vi "ATS_Cards_GBL.vi"() -> ()   [LabVIEW 2010]
doc: "_____AlazarTech, Scope_____\n\nSPecifications of Cards and Pre-set value at Initialization.\n\nCards_Specs: array of specifications of card\n - Name: name of the card\n - Rate: text array of the possible clock rate of the card.\n - Range: text array of the possible input range of the card.\n\nCards_Pre-Set: array of pre-set value for each board."
uses:
  ATS_Card_Spec.ctl
  ATS_Global_4Ch.ctl
  Record.ctl
  Clock.ctl
  ClockSource.ctl
  ClockRate.ctl
  ClockEdge.ctl
  ATS_InputArray.ctl
  InputCtrl.ctl
  Coupling.ctl
  Range.ctl
  Impedance.ctl
  Bandwidth.ctl
  ATS_Trigger_4Ch.ctl
  TriggerOperation.ctl
  ATS_TriggerEngine_4Ch.ctl
  ATS_TriggerSource_4Ch.ctl
  ExtTrigger.ctl
  ExtTrigRange.ctl
  ATS_Global_Specs_Ctrl.ctl
panel:
  in  "Boards_Specs":cluster{"Name":string, "Specifications":T1}[](array[cluster])=[{"Name"="Unknown", "Specifications"={"ClckSource"={"Internal"=TRUE, "External"=TRUE, "Medium Ext."=FALSE, "Slow Ext."=FALSE, "Ext. AC"=FALSE, "Ext. DC"=FALSE, "Ext. (PLL)"=FALSE}, "ClckRate"={"1 kS/s"=TRUE, "2 kS/s"=TRUE, "5 kS/s"=TRUE, "10 kS/s"=TRUE, "20 kS/s"=TRUE, "50 kS/s"=TRUE, "100 kS/s"=TRUE, "200 kS/s"=TRUE, "500 kS/s"=TRUE, "1 MS/s"=TRUE, "2 MS/s"=TRUE, "5 MS/s"=TRUE, "10 MS/s"=TRUE, "20 MS/s"=TRUE, "25 MS/s"=TRUE, "50 MS/s"=TRUE, "100 MS/s"=TRUE, "125 MS/s"=FALSE, "160 MS/s"=FALSE, "180 MS/s"=FALSE, "200 MS/s"=TRUE, "250 MS/s"=FALSE, "500 MS/s"=TRUE, "1 GS/s"=TRUE}, "ClckEdge"={"Rising"=TRUE, "Falling"=TRUE}, "InputCoupling"={"AC"=TRUE, "DC"=TRUE}, "InputRange"={"20mV"=TRUE, "40mV"=TRUE, "50mV"=TRUE, "80mV"=TRUE, "100mV"=TRUE, "200mV"=TRUE, "400mV"=TRUE, "500mV"=TRUE, "800mV"=TRUE, "1 V"=TRUE, "2 V"=TRUE, "4 V"=TRUE, "5 V"=TRUE, "8 V"=TRUE, "10 V"=TRUE, "16 V"=FALSE, "20 V"=TRUE, "40 V"=FALSE, "HiFi"=FALSE, "1.25 V"=FALSE}, "Impedance"={"1M ohms"=TRUE, "50 ohms"=TRUE, "300 ohms"=FALSE}, "Bandwidth"={"Full"=TRUE, "Reduce"=FALSE}, "RangeLim(50)"="20 V", "AsyncDMA"={"OnBoard"=FALSE, "FPGA"=FALSE}, "Memory"={"VerifMem"=FALSE, "HighMem"=FALSE, "Combine"=FALSE, "HighRecord"=FALSE}, "ExtTrigCoupling"={"AC"=TRUE, "DC"=TRUE}, "ExtTrigRange"={"1 V"=TRUE, "5 V"=TRUE, "\nTTL"=FALSE}, "AUX_IO_Trig"={"Trig_Out"=FALSE, "Trig_In"=FALSE}, "AUX_IO_Slope"={"Rising"=FALSE, "Falling"=FALSE}, "MaxPretrig"={"MEM"=0, "FIFO"=0}, "AUX_I/O_Trig"={"OUT_Trigger"=FALSE, "OUT_PACER"=FALSE, "OUT_BUSY"=FALSE, "OUT_CLOCK"=FALSE, "OUT_RESERVED"=FALSE, "OUT_CAPTURE_ALMOST_DONE"=FALSE, "OUT_AUXILIARY"=FALSE, "OUT_SERIAL_DATA"=FALSE, "IN_TRIGGER_ENABLE"=FALSE, "IN_DIGITAL_TRIGGER"=FALSE, "IN_GATE"=FALSE, "IN_CAPTURE_ON_DEMAND"=FALSE, "IN_RESET_TIMESTAMP"=FALSE, "IN_SLOW_EXTERNAL_CLOCK"=FALSE, "INPUT_AUXILIARY"=FALSE, "INPUT_SERIAL_DATA"=FALSE}, "ChannelsPerBoard"=2}}, {"Name"="ATS850", "Specifications"={"ClckSource"={"Internal"=TRUE, "External"=TRUE, "Medium Ext."=FALSE, "Slow Ext."=FALSE, "Ext. AC"=FALSE, "Ext. DC"=FALSE, "Ext. (PLL)"=FALSE}, "ClckRate"={"1 kS/s"=TRUE, "2 kS/s"=TRUE, "5 kS/s"=TRUE, "10 kS/s"=TRUE, "20 kS/s"=TRUE, "50 kS/s"=TRUE, "100 kS/s"=TRUE, "200 kS/s"=TRUE, "500 kS/s"=TRUE, "1 MS/s"=TRUE, "2 MS/s"=TRUE, "5 MS/s"=TRUE, "10 MS/s"=TRUE, "20 MS/s"=FALSE, "25 MS/s"=TRUE, "50 MS/s"=TRUE, "100 MS/s"=FALSE, "125 MS/s"=FALSE, "160 MS/s"=FALSE, "180 MS/s"=FALSE, "200 MS/s"=FALSE, "250 MS/s"=FALSE, "500 MS/s"=FALSE, "1 GS/s"=FALSE}, "ClckEdge"={"Rising"=TRUE, "Falling"=TRUE}, "InputCoupling"={"AC"=TRUE, "DC"=TRUE}, "InputRange"={"20mV"=TRUE, "40mV"=TRUE, "50mV"=TRUE, "80mV"=TRUE, "100mV"=TRUE, "200mV"=TRUE, "400mV"=TRUE, "500mV"=TRUE, "800mV"=TRUE, "1 V"=TRUE, "2 V"=TRUE, "4 V"=TRUE, "5 V"=TRUE, "8 V"=TRUE, "10 V"=TRUE, "16 V"=FALSE, "20 V"=TRUE, "40 V"=FALSE, "HiFi"=FALSE, "1.25 V"=FALSE}, "Impedance"={"1M ohms"=TRUE, "50 ohms"=TRUE, "300 ohms"=FALSE}, "Bandwidth"={"Full"=TRUE, "Reduce"=FALSE}, "RangeLim(50)"="20 V", "AsyncDMA"={"OnBoard"=FALSE, "FPGA"=FALSE}, "Memory"={"VerifMem"=TRUE, "HighMem"=FALSE, "Combine"=FALSE, "HighRecord"=FALSE}, "ExtTrigCoupling"={"AC"=TRUE, "DC"=TRUE}, "ExtTrigRange"={"1 V"=TRUE, "5 V"=TRUE, "\nTTL"=FALSE}, "AUX_IO_Trig"={"Trig_Out"=FALSE, "Trig_In"=FALSE}, "AUX_IO_Slope"={"Rising"=FALSE, "Falling"=FALSE}, "MaxPretrig"={"MEM"=0, "FIFO"=0}, "AUX_I/O_Trig"={"OUT_Trigger"=FALSE, "OUT_PACER"=FALSE, "OUT_BUSY"=FALSE, "OUT_CLOCK"=FALSE, "OUT_RESERVED"=FALSE, "OUT_CAPTURE_ALMOST_DONE"=FALSE, "OUT_AUXILIARY"=FALSE, "OUT_SERIAL_DATA"=FALSE, "IN_TRIGGER_ENABLE"=FALSE, "IN_DIGITAL_TRIGGER"=FALSE, "IN_GATE"=FALSE, "IN_CAPTURE_ON_DEMAND"=FALSE, "IN_RESET_TIMESTAMP"=FALSE, "IN_SLOW_EXTERNAL_CLOCK"=FALSE, "INPUT_AUXILIARY"=FALSE, "INPUT_SERIAL_DATA"=FALSE}, "ChannelsPerBoard"=2}}, {"Name"="ATS310", "Specifications"={"ClckSource"={"Internal"=TRUE, "External"=TRUE, "Medium Ext."=FALSE, "Slow Ext."=FALSE, "Ext. AC"=FALSE, "Ext. DC"=FALSE, "Ext. (PLL)"=FALSE}, "ClckRate"={"1 kS/s"=TRUE, "2 kS/s"=TRUE, "5 kS/s"=TRUE, "10 kS/s"=TRUE, "20 kS/s"=TRUE, "50 kS/s"=TRUE, "100 kS/s"=TRUE, "200 kS/s"=TRUE, "500 kS/s"=TRUE, "1 MS/s"=TRUE, "2 MS/s"=TRUE, "5 MS/s"=TRUE, "10 MS/s"=TRUE, "20 MS/s"=TRUE, "25 MS/s"=FALSE, "50 MS/s"=FALSE, "100 MS/s"=FALSE, "125 MS/s"=FALSE, "160 MS/s"=FALSE, "180 MS/s"=FALSE, "200 MS/s"=FALSE, "250 MS/s"=FALSE, "500 MS/s"=FALSE, "1 GS/s"=FALSE}, "ClckEdge"={"Rising"=TRUE, "Falling"=TRUE}, "InputCoupling"={"AC"=TRUE, "DC"=TRUE}, "InputRange"={"20mV"=FALSE, "40mV"=TRUE, "50mV"=TRUE, "80mV"=TRUE, "100mV"=TRUE, "200mV"=TRUE, "400mV"=TRUE, "500mV"=TRUE, "800mV"=TRUE, "1 V"=TRUE, "2 V"=TRUE, "4 V"=TRUE, "5 V"=TRUE, "8 V"=TRUE, "10 V"=TRUE, "16 V"=FALSE, "20 V"=TRUE, "40 V"=FALSE, "HiFi"=FALSE, "1.25 V"=FALSE}, "Impedance"={"1M ohms"=TRUE, "50 ohms"=TRUE, "300 ohms"=FALSE}, "Bandwidth"={"Full"=TRUE, "Reduce"=FALSE}, "RangeLim(50)"="4 V", "AsyncDMA"={"OnBoard"=FALSE, "FPGA"=FALSE}, "Memory"={"VerifMem"=TRUE, "HighMem"=FALSE, "Combine"=FALSE, "HighRecord"=FALSE}, "ExtTrigCoupling"={"AC"=TRUE, "DC"=TRUE}, "ExtTrigRange"={"1 V"=TRUE, "5 V"=TRUE, "\nTTL"=FALSE}, "AUX_IO_Trig"={"Trig_Out"=FALSE, "Trig_In"=FALSE}, "AUX_IO_Slope"={"Rising"=FALSE, "Falling"=FALSE}, "MaxPretrig"={"MEM"=0, "FIFO"=0}, "AUX_I/O_Trig"={"OUT_Trigger"=FALSE, "OUT_PACER"=FALSE, "OUT_BUSY"=FALSE, "OUT_CLOCK"=FALSE, "OUT_RESERVED"=FALSE, "OUT_CAPTURE_ALMOST_DONE"=FALSE, "OUT_AUXILIARY"=FALSE, "OUT_SERIAL_DATA"=FALSE, "IN_TRIGGER_ENABLE"=FALSE, "IN_DIGITAL_TRIGGER"=FALSE, "IN_GATE"=FALSE, "IN_CAPTURE_ON_DEMAND"=FALSE, "IN_RESET_TIMESTAMP"=FALSE, "IN_SLOW_EXTERNAL_CLOCK"=FALSE, "INPUT_AUXILIARY"=FALSE, "INPUT_SERIAL_DATA"=FALSE}, "ChannelsPerBoard"=2}}, {"Name"="ATS330", "Specifications"={"ClckSource"={"Internal"=TRUE, "External"=TRUE, "Medium Ext."=FALSE, "Slow Ext."=FALSE, "Ext. AC"=FALSE, "Ext. DC"=FALSE, "Ext. (PLL)"=FALSE}, "ClckRate"={"1 kS/s"=TRUE, "2 kS/s"=TRUE, "5 kS/s"=TRUE, "10 kS/s"=TRUE, "20 kS/s"=TRUE, "50 kS/s"=TRUE, "100 kS/s"=TRUE, "200 kS/s"=TRUE, "500 kS/s"=TRUE, "1 MS/s"=TRUE, "2 MS/s"=TRUE, "5 MS/s"=TRUE, "10 MS/s"=TRUE, "20 MS/s"=FALSE, "25 MS/s"=TRUE, "50 MS/s"=TRUE, "100 MS/s"=FALSE, "125 MS/s"=FALSE, "160 MS/s"=FALSE, "180 MS/s"=FALSE, "200 MS/s"=FALSE, "250 MS/s"=FALSE, "500 MS/s"=FALSE, "1 GS/s"=FALSE}, "ClckEdge"={"Rising"=TRUE, "Falling"=TRUE}, "InputCoupling"={"AC"=TRUE, "DC"=TRUE}, "InputRange"={"20mV"=FALSE, "40mV"=TRUE, "50mV"=TRUE, "80mV"=TRUE, "100mV"=TRUE, "200mV"=TRUE, "400mV"=TRUE, "500mV"=TRUE, "800mV"=TRUE, "1 V"=TRUE, "2 V"=TRUE, "4 V"=TRUE, "5 V"=TRUE, "8 V"=TRUE, "10 V"=TRUE, "16 V"=FALSE, "20 V"=TRUE, "40 V"=FALSE, "HiFi"=FALSE, "1.25 V"=FALSE}, "Impedance"={"1M ohms"=TRUE, "50 ohms"=TRUE, "300 ohms"=FALSE}, "Bandwidth"={"Full"=TRUE, "Reduce"=FALSE}, "RangeLim(50)"="4 V", "AsyncDMA"={"OnBoard"=FALSE, "FPGA"=FALSE}, "Memory"={"VerifMem"=TRUE, "HighMem"=FALSE, "Combine"=FALSE, "HighRecord"=FALSE}, "ExtTrigCoupling"={"AC"=TRUE, "DC"=TRUE}, "ExtTrigRange"={"1 V"=TRUE, "5 V"=TRUE, "\nTTL"=FALSE}, "AUX_IO_Trig"={"Trig_Out"=FALSE, "Trig_In"=FALSE}, "AUX_IO_Slope"={"Rising"=FALSE, "Falling"=FALSE}, "MaxPretrig"={"MEM"=0, "FIFO"=0}, "AUX_I/O_Trig"={"OUT_Trigger"=FALSE, "OUT_PACER"=FALSE, "OUT_BUSY"=FALSE, "OUT_CLOCK"=FALSE, "OUT_RESERVED"=FALSE, "OUT_CAPTURE_ALMOST_DONE"=FALSE, "OUT_AUXILIARY"=FALSE, "OUT_SERIAL_DATA"=FALSE, "IN_TRIGGER_ENABLE"=FALSE, "IN_DIGITAL_TRIGGER"=FALSE, "IN_GATE"=FALSE, "IN_CAPTURE_ON_DEMAND"=FALSE, "IN_RESET_TIMESTAMP"=FALSE, "IN_SLOW_EXTERNAL_CLOCK"=FALSE, "INPUT_AUXILIARY"=FALSE, "INPUT_SERIAL_DATA"=FALSE}, "ChannelsPerBoard"=2}}, {"Name"="ATSxx4", "Specifications"={"ClckSource"={"Internal"=TRUE, "External"=TRUE, "Medium Ext."=FALSE, "Slow Ext."=FALSE, "Ext. AC"=FALSE, "Ext. DC"=FALSE, "Ext. (PLL)"=FALSE}, "ClckRate"={"1 kS/s"=TRUE, "2 kS/s"=TRUE, "5 kS/s"=TRUE, "10 kS/s"=TRUE, "20 kS/s"=TRUE, "50 kS/s"=TRUE, "100 kS/s"=TRUE, "200 kS/s"=TRUE, "500 kS/s"=TRUE, "1 MS/s"=TRUE, "2 MS/s"=TRUE, "5 MS/s"=TRUE, "10 MS/s"=TRUE, "20 MS/s"=TRUE, "25 MS/s"=TRUE, "50 MS/s"=TRUE, "100 MS/s"=TRUE, "125 MS/s"=FALSE, "160 MS/s"=FALSE, "180 MS/s"=FALSE, "200 MS/s"=TRUE, "250 MS/s"=FALSE, "500 MS/s"=TRUE, "1 GS/s"=TRUE}, "ClckEdge"={"Rising"=TRUE, "Falling"=TRUE}, "InputCoupling"={"AC"=TRUE, "DC"=TRUE}, "InputRange"={"20mV"=TRUE, "40mV"=TRUE, "50mV"=TRUE, "80mV"=TRUE, "100mV"=TRUE, "200mV"=TRUE, "400mV"=TRUE, "500mV"=TRUE, "800mV"=TRUE, "1 V"=TRUE, "2 V"=TRUE, "4 V"=TRUE, "5 V"=TRUE, "8 V"=TRUE, "10 V"=TRUE, "16 V"=FALSE, "20 V"=TRUE, "40 V"=FALSE, "HiFi"=FALSE, "1.25 V"=FALSE}, "Impedance"={"1M ohms"=TRUE, "50 ohms"=TRUE, "300 ohms"=FALSE}, "Bandwidth"={"Full"=TRUE, "Reduce"=FALSE}, "RangeLim(50)"="20 V", "AsyncDMA"={"OnBoard"=FALSE, "FPGA"=FALSE}, "Memory"={"VerifMem"=FALSE, "HighMem"=FALSE, "Combine"=FALSE, "HighRecord"=FALSE}, "ExtTrigCoupling"={"AC"=TRUE, "DC"=TRUE}, "ExtTrigRange"={"1 V"=TRUE, "5 V"=TRUE, "\nTTL"=FALSE}, "AUX_IO_Trig"={"Trig_Out"=FALSE, "Trig_In"=FALSE}, "AUX_IO_Slope"={"Rising"=FALSE, "Falling"=FALSE}, "MaxPretrig"={"MEM"=0, "FIFO"=0}, "AUX_I/O_Trig"={"OUT_Trigger"=FALSE, "OUT_PACER"=FALSE, "OUT_BUSY"=FALSE, "OUT_CLOCK"=FALSE, "OUT_RESERVED"=FALSE, "OUT_CAPTURE_ALMOST_DONE"=FALSE, "OUT_AUXILIARY"=FALSE, "OUT_SERIAL_DATA"=FALSE, "IN_TRIGGER_ENABLE"=FALSE, "IN_DIGITAL_TRIGGER"=FALSE, "IN_GATE"=FALSE, "IN_CAPTURE_ON_DEMAND"=FALSE, "IN_RESET_TIMESTAMP"=FALSE, "IN_SLOW_EXTERNAL_CLOCK"=FALSE, "INPUT_AUXILIARY"=FALSE, "INPUT_SERIAL_DATA"=FALSE}, "ChannelsPerBoard"=2}}, {"Name"="ATSxx5", "Specifications"={"ClckSource"={"Internal"=TRUE, "External"=TRUE, "Medium Ext."=FALSE, "Slow Ext."=FALSE, "Ext. AC"=FALSE, "Ext. DC"=FALSE, "Ext. (PLL)"=FALSE}, "ClckRate"={"1 kS/s"=TRUE, "2 kS/s"=TRUE, "5 kS/s"=TRUE, "10 kS/s"=TRUE, "20 kS/s"=TRUE, "50 kS/s"=TRUE, "100 kS/s"=TRUE, "200 kS/s"=TRUE, "500 kS/s"=TRUE, "1 MS/s"=TRUE, "2 MS/s"=TRUE, "5 MS/s"=TRUE, "10 MS/s"=TRUE, "20 MS/s"=TRUE, "25 MS/s"=TRUE, "50 MS/s"=TRUE, "100 MS/s"=TRUE, "125 MS/s"=FALSE, "160 MS/s"=FALSE, "180 MS/s"=FALSE, "200 MS/s"=TRUE, "250 MS/s"=FALSE, "500 MS/s"=TRUE, "1 GS/s"=TRUE}, "ClckEdge"={"Rising"=TRUE, "Falling"=TRUE}, "InputCoupling"={"AC"=TRUE, "DC"=TRUE}, "InputRange"={"20mV"=TRUE, "40mV"=TRUE, "50mV"=TRUE, "80mV"=TRUE, "100mV"=TRUE, "200mV"=TRUE, "400mV"=TRUE, "500mV"=TRUE, "800mV"=TRUE, "1 V"=TRUE, "2 V"=TRUE, "4 V"=TRUE, "5 V"=TRUE, "8 V"=TRUE, "10 V"=TRUE, "16 V"=FALSE, "20 V"=TRUE, "40 V"=FALSE, "HiFi"=FALSE, "1.25 V"=FALSE}, "Impedance"={"1M ohms"=TRUE, "50 ohms"=TRUE, "300 ohms"=FALSE}, "Bandwidth"={"Full"=TRUE, "Reduce"=FALSE}, "RangeLim(50)"="20 V", "AsyncDMA"={"OnBoard"=FALSE, "FPGA"=FALSE}, "Memory"={"VerifMem"=FALSE, "HighMem"=FALSE, "Combine"=FALSE, "HighRecord"=FALSE}, "ExtTrigCoupling"={"AC"=TRUE, "DC"=TRUE}, "ExtTrigRange"={"1 V"=TRUE, "5 V"=TRUE, "\nTTL"=FALSE}, "AUX_IO_Trig"={"Trig_Out"=FALSE, "Trig_In"=FALSE}, "AUX_IO_Slope"={"Rising"=FALSE, "Falling"=FALSE}, "MaxPretrig"={"MEM"=0, "FIFO"=0}, "AUX_I/O_Trig"={"OUT_Trigger"=FALSE, "OUT_PACER"=FALSE, "OUT_BUSY"=FALSE, "OUT_CLOCK"=FALSE, "OUT_RESERVED"=FALSE, "OUT_CAPTURE_ALMOST_DONE"=FALSE, "OUT_AUXILIARY"=FALSE, "OUT_SERIAL_DATA"=FALSE, "IN_TRIGGER_ENABLE"=FALSE, "IN_DIGITAL_TRIGGER"=FALSE, "IN_GATE"=FALSE, "IN_CAPTURE_ON_DEMAND"=FALSE, "IN_RESET_TIMESTAMP"=FALSE, "IN_SLOW_EXTERNAL_CLOCK"=FALSE, "INPUT_AUXILIARY"=FALSE, "INPUT_SERIAL_DATA"=FALSE}, "ChannelsPerBoard"=2}}, {"Name"="ATS460", "Specifications"={"ClckSource"={"Internal"=TRUE, "External"=TRUE, "Medium Ext."=TRUE, "Slow Ext."=TRUE, "Ext. AC"=FALSE, "Ext. DC"=FALSE, "Ext. (PLL)"=FALSE}, "ClckRate"={"1 kS/s"=FALSE, "2 kS/s"=FALSE, "5 kS/s"=FALSE, "10 kS/s"=TRUE, "20 kS/s"=TRUE, "50 kS/s"=TRUE, "100 kS/s"=TRUE, "200 kS/s"=TRUE, "500 kS/s"=TRUE, "1 MS/s"=TRUE, "2 MS/s"=TRUE, "5 MS/s"=TRUE, "10 MS/s"=TRUE, "20 MS/s"=TRUE, "25 MS/s"=FALSE, "50 MS/s"=TRUE, "100 MS/s"=TRUE, "125 MS/s"=TRUE, "160 MS/s"=FALSE, "180 MS/s"=FALSE, "200 MS/s"=FALSE, "250 MS/s"=FALSE, "500 MS/s"=FALSE, "1 GS/s"=FALSE}, "ClckEdge"={"Rising"=TRUE, "Falling"=TRUE}, "InputCoupling"={"AC"=TRUE, "DC"=TRUE}, "InputRange"={"20mV"=TRUE, "40mV"=TRUE, "50mV"=TRUE, "80mV"=TRUE, "100mV"=TRUE, "200mV"=TRUE, "400mV"=TRUE, "500mV"=TRUE, "800mV"=TRUE, "1 V"=TRUE, "2 V"=TRUE, "4 V"=TRUE, "5 V"=TRUE, "8 V"=TRUE, "10 V"=TRUE, "16 V"=FALSE, "20 V"=FALSE, "40 V"=FALSE, "HiFi"=TRUE, "1.25 V"=FALSE}, "Impedance"={"1M ohms"=TRUE, "50 ohms"=TRUE, "300 ohms"=FALSE}, "Bandwidth"={"Full"=TRUE, "Reduce"=TRUE}, "RangeLim(50)"="4 V", "AsyncDMA"={"OnBoard"=TRUE, "FPGA"=FALSE}, "Memory"={"VerifMem"=FALSE, "HighMem"=TRUE, "Combine"=FALSE, "HighRecord"=TRUE}, "ExtTrigCoupling"={"AC"=TRUE, "DC"=TRUE}, "ExtTrigRange"={"1 V"=TRUE, "5 V"=TRUE, "\nTTL"=FALSE}, "AUX_IO_Trig"={"Trig_Out"=FALSE, "Trig_In"=FALSE}, "AUX_IO_Slope"={"Rising"=FALSE, "Falling"=FALSE}, "MaxPretrig"={"MEM"=305419896, "FIFO"=0}, "AUX_I/O_Trig"={"OUT_Trigger"=FALSE, "OUT_PACER"=FALSE, "OUT_BUSY"=FALSE, "OUT_CLOCK"=FALSE, "OUT_RESERVED"=FALSE, "OUT_CAPTURE_ALMOST_DONE"=FALSE, "OUT_AUXILIARY"=FALSE, "OUT_SERIAL_DATA"=FALSE, "IN_TRIGGER_ENABLE"=FALSE, "IN_DIGITAL_TRIGGER"=FALSE, "IN_GATE"=FALSE, "IN_CAPTURE_ON_DEMAND"=FALSE, "IN_RESET_TIMESTAMP"=FALSE, "IN_SLOW_EXTERNAL_CLOCK"=FALSE, "INPUT_AUXILIARY"=FALSE, "INPUT_SERIAL_DATA"=FALSE}, "ChannelsPerBoard"=2}}, {"Name"="ATS660", "Specifications"={"ClckSource"={"Internal"=TRUE, "External"=TRUE, "Medium Ext."=FALSE, "Slow Ext."=TRUE, "Ext. AC"=TRUE, "Ext. DC"=TRUE, "Ext. (PLL)"=TRUE}, "ClckRate"={"1 kS/s"=TRUE, "2 kS/s"=TRUE, "5 kS/s"=TRUE, "10 kS/s"=TRUE, "20 kS/s"=TRUE, "50 kS/s"=TRUE, "100 kS/s"=TRUE, "200 kS/s"=TRUE, "500 kS/s"=TRUE, "1 MS/s"=TRUE, "2 MS/s"=TRUE, "5 MS/s"=TRUE, "10 MS/s"=TRUE, "20 MS/s"=TRUE, "25 MS/s"=FALSE, "50 MS/s"=TRUE, "100 MS/s"=TRUE, "125 MS/s"=TRUE, "160 MS/s"=FALSE, "180 MS/s"=FALSE, "200 MS/s"=FALSE, "250 MS/s"=FALSE, "500 MS/s"=FALSE, "1 GS/s"=FALSE}, "ClckEdge"={"Rising"=TRUE, "Falling"=TRUE}, "InputCoupling"={"AC"=TRUE, "DC"=TRUE}, "InputRange"={"20mV"=FALSE, "40mV"=FALSE, "50mV"=FALSE, "80mV"=FALSE, "100mV"=FALSE, "200mV"=TRUE, "400mV"=TRUE, "500mV"=FALSE, "800mV"=TRUE, "1 V"=FALSE, "2 V"=TRUE, "4 V"=TRUE, "5 V"=FALSE, "8 V"=TRUE, "10 V"=FALSE, "16 V"=TRUE, "20 V"=FALSE, "40 V"=FALSE, "HiFi"=FALSE, "1.25 V"=FALSE}, "Impedance"={"1M ohms"=TRUE, "50 ohms"=TRUE, "300 ohms"=FALSE}, "Bandwidth"={"Full"=TRUE, "Reduce"=TRUE}, "RangeLim(50)"="4 V", "AsyncDMA"={"OnBoard"=TRUE, "FPGA"=FALSE}, "Memory"={"VerifMem"=FALSE, "HighMem"=TRUE, "Combine"=FALSE, "HighRecord"=TRUE}, "ExtTrigCoupling"={"AC"=TRUE, "DC"=TRUE}, "ExtTrigRange"={"1 V"=TRUE, "5 V"=TRUE, "\nTTL"=FALSE}, "AUX_IO_Trig"={"Trig_Out"=FALSE, "Trig_In"=FALSE}, "AUX_IO_Slope"={"Rising"=FALSE, "Falling"=FALSE}, "MaxPretrig"={"MEM"=8386560, "FIFO"=0}, "AUX_I/O_Trig"={"OUT_Trigger"=FALSE, "OUT_PACER"=FALSE, "OUT_BUSY"=FALSE, "OUT_CLOCK"=FALSE, "OUT_RESERVED"=FALSE, "OUT_CAPTURE_ALMOST_DONE"=FALSE, "OUT_AUXILIARY"=FALSE, "OUT_SERIAL_DATA"=FALSE, "IN_TRIGGER_ENABLE"=FALSE, "IN_DIGITAL_TRIGGER"=FALSE, "IN_GATE"=FALSE, "IN_CAPTURE_ON_DEMAND"=FALSE, "IN_RESET_TIMESTAMP"=FALSE, "IN_SLOW_EXTERNAL_CLOCK"=FALSE, "INPUT_AUXILIARY"=FALSE, "INPUT_SERIAL_DATA"=FALSE}, "ChannelsPerBoard"=2}}, {"Name"="ATS860", "Specifications"={"ClckSource"={"Internal"=TRUE, "External"=TRUE, "Medium Ext."=FALSE, "Slow Ext."=FALSE, "Ext. AC"=FALSE, "Ext. DC"=FALSE, "Ext. (PLL)"=FALSE}, "ClckRate"={"1 kS/s"=TRUE, "2 kS/s"=TRUE, "5 kS/s"=TRUE, "10 kS/s"=TRUE, "20 kS/s"=TRUE, "50 kS/s"=TRUE, "100 kS/s"=TRUE, "200 kS/s"=TRUE, "500 kS/s"=TRUE, "1 MS/s"=TRUE, "2 MS/s"=TRUE, "5 MS/s"=TRUE, "10 MS/s"=TRUE, "20 MS/s"=FALSE, "25 MS/s"=TRUE, "50 MS/s"=TRUE, "100 MS/s"=FALSE, "125 MS/s"=TRUE, "160 MS/s"=FALSE, "180 MS/s"=FALSE, "200 MS/s"=FALSE, "250 MS/s"=TRUE, "500 MS/s"=FALSE, "1 GS/s"=FALSE}, "ClckEdge"={"Rising"=TRUE, "Falling"=TRUE}, "InputCoupling"={"AC"=TRUE, "DC"=TRUE}, "InputRange"={"20mV"=TRUE, "40mV"=TRUE, "50mV"=TRUE, "80mV"=TRUE, "100mV"=TRUE, "200mV"=TRUE, "400mV"=TRUE, "500mV"=TRUE, "800mV"=TRUE, "1 V"=TRUE, "2 V"=TRUE, "4 V"=TRUE, "5 V"=TRUE, "8 V"=TRUE, "10 V"=TRUE, "16 V"=FALSE, "20 V"=FALSE, "40 V"=FALSE, "HiFi"=FALSE, "1.25 V"=FALSE}, "Impedance"={"1M ohms"=TRUE, "50 ohms"=TRUE, "300 ohms"=FALSE}, "Bandwidth"={"Full"=TRUE, "Reduce"=TRUE}, "RangeLim(50)"="4 V", "AsyncDMA"={"OnBoard"=TRUE, "FPGA"=FALSE}, "Memory"={"VerifMem"=FALSE, "HighMem"=TRUE, "Combine"=FALSE, "HighRecord"=TRUE}, "ExtTrigCoupling"={"AC"=TRUE, "DC"=TRUE}, "ExtTrigRange"={"1 V"=TRUE, "5 V"=TRUE, "\nTTL"=FALSE}, "AUX_IO_Trig"={"Trig_Out"=FALSE, "Trig_In"=FALSE}, "AUX_IO_Slope"={"Rising"=FALSE, "Falling"=FALSE}, "MaxPretrig"={"MEM"=0, "FIFO"=0}, "AUX_I/O_Trig"={"OUT_Trigger"=FALSE, "OUT_PACER"=FALSE, "OUT_BUSY"=FALSE, "OUT_CLOCK"=FALSE, "OUT_RESERVED"=FALSE, "OUT_CAPTURE_ALMOST_DONE"=FALSE, "OUT_AUXILIARY"=FALSE, "OUT_SERIAL_DATA"=FALSE, "IN_TRIGGER_ENABLE"=FALSE, "IN_DIGITAL_TRIGGER"=FALSE, "IN_GATE"=FALSE, "IN_CAPTURE_ON_DEMAND"=FALSE, "IN_RESET_TIMESTAMP"=FALSE, "IN_SLOW_EXTERNAL_CLOCK"=FALSE, "INPUT_AUXILIARY"=FALSE, "INPUT_SERIAL_DATA"=FALSE}, "ChannelsPerBoard"=2}}, {"Name"="Unknown", "Specifications"={"ClckSource"={"Internal"=TRUE, "External"=TRUE, "Medium Ext."=FALSE, "Slow Ext."=FALSE, "Ext. AC"=FALSE, "Ext. DC"=FALSE, "Ext. (PLL)"=FALSE}, "ClckRate"={"1 kS/s"=TRUE, "2 kS/s"=TRUE, "5 kS/s"=TRUE, "10 kS/s"=TRUE, "20 kS/s"=TRUE, "50 kS/s"=TRUE, "100 kS/s"=TRUE, "200 kS/s"=TRUE, "500 kS/s"=TRUE, "1 MS/s"=TRUE, "2 MS/s"=TRUE, "5 MS/s"=TRUE, "10 MS/s"=TRUE, "20 MS/s"=TRUE, "25 MS/s"=FALSE, "50 MS/s"=TRUE, "100 MS/s"=TRUE, "125 MS/s"=TRUE, "160 MS/s"=FALSE, "180 MS/s"=FALSE, "200 MS/s"=FALSE, "250 MS/s"=FALSE, "500 MS/s"=FALSE, "1 GS/s"=FALSE}, "ClckEdge"={"Rising"=TRUE, "Falling"=TRUE}, "InputCoupling"={"AC"=TRUE, "DC"=TRUE}, "InputRange"={"20mV"=FALSE, "40mV"=FALSE, "50mV"=FALSE, "80mV"=FALSE, "100mV"=FALSE, "200mV"=TRUE, "400mV"=TRUE, "500mV"=FALSE, "800mV"=TRUE, "1 V"=FALSE, "2 V"=TRUE, "4 V"=TRUE, "5 V"=FALSE, "8 V"=TRUE, "10 V"=FALSE, "16 V"=TRUE, "20 V"=FALSE, "40 V"=FALSE, "HiFi"=FALSE, "1.25 V"=FALSE}, "Impedance"={"1M ohms"=TRUE, "50 ohms"=TRUE, "300 ohms"=FALSE}, "Bandwidth"={"Full"=TRUE, "Reduce"=TRUE}, "RangeLim(50)"="4 V", "AsyncDMA"={"OnBoard"=FALSE, "FPGA"=FALSE}, "Memory"={"VerifMem"=FALSE, "HighMem"=FALSE, "Combine"=FALSE, "HighRecord"=FALSE}, "ExtTrigCoupling"={"AC"=TRUE, "DC"=TRUE}, "ExtTrigRange"={"1 V"=TRUE, "5 V"=TRUE, "\nTTL"=FALSE}, "AUX_IO_Trig"={"Trig_Out"=FALSE, "Trig_In"=FALSE}, "AUX_IO_Slope"={"Rising"=FALSE, "Falling"=FALSE}, "MaxPretrig"={"MEM"=0, "FIFO"=0}, "AUX_I/O_Trig"={"OUT_Trigger"=FALSE, "OUT_PACER"=FALSE, "OUT_BUSY"=FALSE, "OUT_CLOCK"=FALSE, "OUT_RESERVED"=FALSE, "OUT_CAPTURE_ALMOST_DONE"=FALSE, "OUT_AUXILIARY"=FALSE, "OUT_SERIAL_DATA"=FALSE, "IN_TRIGGER_ENABLE"=FALSE, "IN_DIGITAL_TRIGGER"=FALSE, "IN_GATE"=FALSE, "IN_CAPTURE_ON_DEMAND"=FALSE, "IN_RESET_TIMESTAMP"=FALSE, "IN_SLOW_EXTERNAL_CLOCK"=FALSE, "INPUT_AUXILIARY"=FALSE, "INPUT_SERIAL_DATA"=FALSE}, "ChannelsPerBoard"=2}}, {"Name"="Unknown", "Specifications"={"ClckSource"={"Internal"=TRUE, "External"=TRUE, "Medium Ext."=FALSE, "Slow Ext."=FALSE, "Ext. AC"=FALSE, "Ext. DC"=FALSE, "Ext. (PLL)"=FALSE}, "ClckRate"={"1 kS/s"=TRUE, "2 kS/s"=TRUE, "5 kS/s"=TRUE, "10 kS/s"=TRUE, "20 kS/s"=TRUE, "50 kS/s"=TRUE, "100 kS/s"=TRUE, "200 kS/s"=TRUE, "500 kS/s"=TRUE, "1 MS/s"=TRUE, "2 MS/s"=TRUE, "5 MS/s"=TRUE, "10 MS/s"=TRUE, "20 MS/s"=TRUE, "25 MS/s"=FALSE, "50 MS/s"=TRUE, "100 MS/s"=TRUE, "125 MS/s"=TRUE, "160 MS/s"=FALSE, "180 MS/s"=FALSE, "200 MS/s"=FALSE, "250 MS/s"=FALSE, "500 MS/s"=FALSE, "1 GS/s"=FALSE}, "ClckEdge"={"Rising"=TRUE, "Falling"=TRUE}, "InputCoupling"={"AC"=TRUE, "DC"=TRUE}, "InputRange"={"20mV"=FALSE, "40mV"=FALSE, "50mV"=FALSE, "80mV"=FALSE, "100mV"=FALSE, "200mV"=TRUE, "400mV"=TRUE, "500mV"=FALSE, "800mV"=TRUE, "1 V"=FALSE, "2 V"=TRUE, "4 V"=TRUE, "5 V"=FALSE, "8 V"=TRUE, "10 V"=FALSE, "16 V"=TRUE, "20 V"=FALSE, "40 V"=FALSE, "HiFi"=FALSE, "1.25 V"=FALSE}, "Impedance"={"1M ohms"=TRUE, "50 ohms"=TRUE, "300 ohms"=FALSE}, "Bandwidth"={"Full"=TRUE, "Reduce"=TRUE}, "RangeLim(50)"="4 V", "AsyncDMA"={"OnBoard"=FALSE, "FPGA"=FALSE}, "Memory"={"VerifMem"=FALSE, "HighMem"=FALSE, "Combine"=FALSE, "HighRecord"=FALSE}, "ExtTrigCoupling"={"AC"=TRUE, "DC"=TRUE}, "ExtTrigRange"={"1 V"=TRUE, "5 V"=TRUE, "\nTTL"=FALSE}, "AUX_IO_Trig"={"Trig_Out"=FALSE, "Trig_In"=FALSE}, "AUX_IO_Slope"={"Rising"=FALSE, "Falling"=FALSE}, "MaxPretrig"={"MEM"=0, "FIFO"=0}, "AUX_I/O_Trig"={"OUT_Trigger"=FALSE, "OUT_PACER"=FALSE, "OUT_BUSY"=FALSE, "OUT_CLOCK"=FALSE, "OUT_RESERVED"=FALSE, "OUT_CAPTURE_ALMOST_DONE"=FALSE, "OUT_AUXILIARY"=FALSE, "OUT_SERIAL_DATA"=FALSE, "IN_TRIGGER_ENABLE"=FALSE, "IN_DIGITAL_TRIGGER"=FALSE, "IN_GATE"=FALSE, "IN_CAPTURE_ON_DEMAND"=FALSE, "IN_RESET_TIMESTAMP"=FALSE, "IN_SLOW_EXTERNAL_CLOCK"=FALSE, "INPUT_AUXILIARY"=FALSE, "INPUT_SERIAL_DATA"=FALSE}, "ChannelsPerBoard"=2}}, {"Name"="ATS9462", "Specifications"={"ClckSource"={"Internal"=TRUE, "External"=TRUE, "Medium Ext."=FALSE, "Slow Ext."=TRUE, "Ext. AC"=FALSE, "Ext. DC"=TRUE, "Ext. (PLL)"=TRUE}, "ClckRate"={"1 kS/s"=TRUE, "2 kS/s"=TRUE, "5 kS/s"=TRUE, "10 kS/s"=TRUE, "20 kS/s"=TRUE, "50 kS/s"=TRUE, "100 kS/s"=TRUE, "200 kS/s"=TRUE, "500 kS/s"=TRUE, "1 MS/s"=TRUE, "2 MS/s"=TRUE, "5 MS/s"=TRUE, "10 MS/s"=TRUE, "20 MS/s"=TRUE, "25 MS/s"=FALSE, "50 MS/s"=TRUE, "100 MS/s"=TRUE, "125 MS/s"=TRUE, "160 MS/s"=TRUE, "180 MS/s"=TRUE, "200 MS/s"=FALSE, "250 MS/s"=FALSE, "500 MS/s"=FALSE, "1 GS/s"=FALSE}, "ClckEdge"={"Rising"=TRUE, "Falling"=TRUE}, "InputCoupling"={"AC"=TRUE, "DC"=TRUE}, "InputRange"={"20mV"=FALSE, "40mV"=FALSE, "50mV"=FALSE, "80mV"=FALSE, "100mV"=FALSE, "200mV"=TRUE, "400mV"=TRUE, "500mV"=FALSE, "800mV"=TRUE, "1 V"=FALSE, "2 V"=TRUE, "4 V"=TRUE, "5 V"=FALSE, "8 V"=TRUE, "10 V"=FALSE, "16 V"=TRUE, "20 V"=FALSE, "40 V"=FALSE, "HiFi"=FALSE, "1.25 V"=FALSE}, "Impedance"={"1M ohms"=TRUE, "50 ohms"=TRUE, "300 ohms"=FALSE}, "Bandwidth"={"Full"=TRUE, "Reduce"=TRUE}, "RangeLim(50)"="4 V", "AsyncDMA"={"OnBoard"=TRUE, "FPGA"=TRUE}, "Memory"={"VerifMem"=FALSE, "HighMem"=TRUE, "Combine"=FALSE, "HighRecord"=TRUE}, "ExtTrigCoupling"={"AC"=TRUE, "DC"=TRUE}, "ExtTrigRange"={"1 V"=TRUE, "5 V"=TRUE, "\nTTL"=FALSE}, "AUX_IO_Trig"={"Trig_Out"=TRUE, "Trig_In"=TRUE}, "AUX_IO_Slope"={"Rising"=TRUE, "Falling"=TRUE}, "MaxPretrig"={"MEM"=0, "FIFO"=0}, "AUX_I/O_Trig"={"OUT_Trigger"=TRUE, "OUT_PACER"=FALSE, "OUT_BUSY"=FALSE, "OUT_CLOCK"=FALSE, "OUT_RESERVED"=FALSE, "OUT_CAPTURE_ALMOST_DONE"=FALSE, "OUT_AUXILIARY"=FALSE, "OUT_SERIAL_DATA"=FALSE, "IN_TRIGGER_ENABLE"=TRUE, "IN_DIGITAL_TRIGGER"=TRUE, "IN_GATE"=FALSE, "IN_CAPTURE_ON_DEMAND"=FALSE, "IN_RESET_TIMESTAMP"=FALSE, "IN_SLOW_EXTERNAL_CLOCK"=FALSE, "INPUT_AUXILIARY"=FALSE, "INPUT_SERIAL_DATA"=FALSE}, "ChannelsPerBoard"=2}}, {"Name"="Unknown", "Specifications"={"ClckSource"={"Internal"=TRUE, "External"=TRUE, "Medium Ext."=FALSE, "Slow Ext."=FALSE, "Ext. AC"=FALSE, "Ext. DC"=FALSE, "Ext. (PLL)"=FALSE}, "ClckRate"={"1 kS/s"=TRUE, "2 kS/s"=TRUE, "5 kS/s"=TRUE, "10 kS/s"=TRUE, "20 kS/s"=TRUE, "50 kS/s"=TRUE, "100 kS/s"=TRUE, "200 kS/s"=TRUE, "500 kS/s"=TRUE, "1 MS/s"=TRUE, "2 MS/s"=TRUE, "5 MS/s"=TRUE, "10 MS/s"=TRUE, "20 MS/s"=TRUE, "25 MS/s"=FALSE, "50 MS/s"=TRUE, "100 MS/s"=TRUE, "125 MS/s"=TRUE, "160 MS/s"=FALSE, "180 MS/s"=FALSE, "200 MS/s"=FALSE, "250 MS/s"=FALSE, "500 MS/s"=FALSE, "1 GS/s"=FALSE}, "ClckEdge"={"Rising"=TRUE, "Falling"=TRUE}, "InputCoupling"={"AC"=TRUE, "DC"=TRUE}, "InputRange"={"20mV"=FALSE, "40mV"=FALSE, "50mV"=FALSE, "80mV"=FALSE, "100mV"=FALSE, "200mV"=TRUE, "400mV"=TRUE, "500mV"=FALSE, "800mV"=TRUE, "1 V"=FALSE, "2 V"=TRUE, "4 V"=TRUE, "5 V"=FALSE, "8 V"=TRUE, "10 V"=FALSE, "16 V"=TRUE, "20 V"=FALSE, "40 V"=FALSE, "HiFi"=FALSE, "1.25 V"=FALSE}, "Impedance"={"1M ohms"=TRUE, "50 ohms"=TRUE, "300 ohms"=FALSE}, "Bandwidth"={"Full"=TRUE, "Reduce"=TRUE}, "RangeLim(50)"="4 V", "AsyncDMA"={"OnBoard"=FALSE, "FPGA"=FALSE}, "Memory"={"VerifMem"=FALSE, "HighMem"=FALSE, "Combine"=FALSE, "HighRecord"=FALSE}, "ExtTrigCoupling"={"AC"=TRUE, "DC"=TRUE}, "ExtTrigRange"={"1 V"=TRUE, "5 V"=TRUE, "\nTTL"=FALSE}, "AUX_IO_Trig"={"Trig_Out"=FALSE, "Trig_In"=FALSE}, "AUX_IO_Slope"={"Rising"=FALSE, "Falling"=FALSE}, "MaxPretrig"={"MEM"=0, "FIFO"=0}, "AUX_I/O_Trig"={"OUT_Trigger"=FALSE, "OUT_PACER"=FALSE, "OUT_BUSY"=FALSE, "OUT_CLOCK"=FALSE, "OUT_RESERVED"=FALSE, "OUT_CAPTURE_ALMOST_DONE"=FALSE, "OUT_AUXILIARY"=FALSE, "OUT_SERIAL_DATA"=FALSE, "IN_TRIGGER_ENABLE"=FALSE, "IN_DIGITAL_TRIGGER"=FALSE, "IN_GATE"=FALSE, "IN_CAPTURE_ON_DEMAND"=FALSE, "IN_RESET_TIMESTAMP"=FALSE, "IN_SLOW_EXTERNAL_CLOCK"=FALSE, "INPUT_AUXILIARY"=FALSE, "INPUT_SERIAL_DATA"=FALSE}, "ChannelsPerBoard"=2}}, {"Name"="ATS9870", "Specifications"={"ClckSource"={"Internal"=TRUE, "External"=TRUE, "Medium Ext."=FALSE, "Slow Ext."=FALSE, "Ext. AC"=TRUE, "Ext. DC"=TRUE, "Ext. (PLL)"=TRUE}, "ClckRate"={"1 kS/s"=TRUE, "2 kS/s"=TRUE, "5 kS/s"=TRUE, "10 kS/s"=TRUE, "20 kS/s"=TRUE, "50 kS/s"=TRUE, "100 kS/s"=TRUE, "200 kS/s"=TRUE, "500 kS/s"=TRUE, "1 MS/s"=TRUE, "2 MS/s"=TRUE, "5 MS/s"=TRUE, "10 MS/s"=TRUE, "20 MS/s"=TRUE, "25 MS/s"=FALSE, "50 MS/s"=TRUE, "100 MS/s"=TRUE, "125 MS/s"=FALSE, "160 MS/s"=FALSE, "180 MS/s"=FALSE, "200 MS/s"=FALSE, "250 MS/s"=TRUE, "500 MS/s"=TRUE, "1 GS/s"=TRUE}, "ClckEdge"={"Rising"=TRUE, "Falling"=TRUE}, "InputCoupling"={"AC"=TRUE, "DC"=TRUE}, "InputRange"={"20mV"=FALSE, "40mV"=TRUE, "50mV"=FALSE, "80mV"=FALSE, "100mV"=TRUE, "200mV"=TRUE, "400mV"=TRUE, "500mV"=FALSE, "800mV"=FALSE, "1 V"=TRUE, "2 V"=TRUE, "4 V"=TRUE, "5 V"=FALSE, "8 V"=FALSE, "10 V"=FALSE, "16 V"=FALSE, "20 V"=FALSE, "40 V"=FALSE, "HiFi"=FALSE, "1.25 V"=FALSE}, "Impedance"={"1M ohms"=FALSE, "50 ohms"=TRUE, "300 ohms"=FALSE}, "Bandwidth"={"Full"=TRUE, "Reduce"=TRUE}, "RangeLim(50)"="4 V", "AsyncDMA"={"OnBoard"=TRUE, "FPGA"=TRUE}, "Memory"={"VerifMem"=FALSE, "HighMem"=TRUE, "Combine"=FALSE, "HighRecord"=TRUE}, "ExtTrigCoupling"={"AC"=FALSE, "DC"=TRUE}, "ExtTrigRange"={"1 V"=TRUE, "5 V"=TRUE, "\nTTL"=FALSE}, "AUX_IO_Trig"={"Trig_Out"=TRUE, "Trig_In"=TRUE}, "AUX_IO_Slope"={"Rising"=TRUE, "Falling"=TRUE}, "MaxPretrig"={"MEM"=0, "FIFO"=0}, "AUX_I/O_Trig"={"OUT_Trigger"=TRUE, "OUT_PACER"=FALSE, "OUT_BUSY"=FALSE, "OUT_CLOCK"=FALSE, "OUT_RESERVED"=FALSE, "OUT_CAPTURE_ALMOST_DONE"=FALSE, "OUT_AUXILIARY"=FALSE, "OUT_SERIAL_DATA"=FALSE, "IN_TRIGGER_ENABLE"=TRUE, "IN_DIGITAL_TRIGGER"=TRUE, "IN_GATE"=FALSE, "IN_CAPTURE_ON_DEMAND"=FALSE, "IN_RESET_TIMESTAMP"=FALSE, "IN_SLOW_EXTERNAL_CLOCK"=FALSE, "INPUT_AUXILIARY"=FALSE, "INPUT_SERIAL_DATA"=FALSE}, "ChannelsPerBoard"=2}}, {"Name"="ATS9350", "Specifications"={"ClckSource"={"Internal"=TRUE, "External"=TRUE, "Medium Ext."=FALSE, "Slow Ext."=TRUE, "Ext. AC"=FALSE, "Ext. DC"=FALSE, "Ext. (PLL)"=TRUE}, "ClckRate"={"1 kS/s"=TRUE, "2 kS/s"=TRUE, "5 kS/s"=TRUE, "10 kS/s"=TRUE, "20 kS/s"=TRUE, "50 kS/s"=TRUE, "100 kS/s"=TRUE, "200 kS/s"=TRUE, "500 kS/s"=TRUE, "1 MS/s"=TRUE, "2 MS/s"=TRUE, "5 MS/s"=TRUE, "10 MS/s"=TRUE, "20 MS/s"=TRUE, "25 MS/s"=FALSE, "50 MS/s"=TRUE, "100 MS/s"=TRUE, "125 MS/s"=FALSE, "160 MS/s"=FALSE, "180 MS/s"=FALSE, "200 MS/s"=FALSE, "250 MS/s"=TRUE, "500 MS/s"=TRUE, "1 GS/s"=FALSE}, "ClckEdge"={"Rising"=TRUE, "Falling"=TRUE}, "InputCoupling"={"AC"=TRUE, "DC"=TRUE}, "InputRange"={"20mV"=FALSE, "40mV"=TRUE, "50mV"=FALSE, "80mV"=FALSE, "100mV"=TRUE, "200mV"=TRUE, "400mV"=TRUE, "500mV"=FALSE, "800mV"=FALSE, "1 V"=TRUE, "2 V"=TRUE, "4 V"=TRUE, "5 V"=FALSE, "8 V"=FALSE, "10 V"=FALSE, "16 V"=FALSE, "20 V"=FALSE, "40 V"=FALSE, "HiFi"=FALSE, "1.25 V"=FALSE}, "Impedance"={"1M ohms"=FALSE, "50 ohms"=TRUE, "300 ohms"=FALSE}, "Bandwidth"={"Full"=TRUE, "Reduce"=FALSE}, "RangeLim(50)"="4 V", "AsyncDMA"={"OnBoard"=TRUE, "FPGA"=FALSE}, "Memory"={"VerifMem"=FALSE, "HighMem"=TRUE, "Combine"=FALSE, "HighRecord"=TRUE}, "ExtTrigCoupling"={"AC"=TRUE, "DC"=TRUE}, "ExtTrigRange"={"1 V"=TRUE, "5 V"=TRUE, "\nTTL"=TRUE}, "AUX_IO_Trig"={"Trig_Out"=TRUE, "Trig_In"=TRUE}, "AUX_IO_Slope"={"Rising"=TRUE, "Falling"=TRUE}, "MaxPretrig"={"MEM"=0, "FIFO"=0}, "AUX_I/O_Trig"={"OUT_Trigger"=TRUE, "OUT_PACER"=FALSE, "OUT_BUSY"=FALSE, "OUT_CLOCK"=FALSE, "OUT_RESERVED"=FALSE, "OUT_CAPTURE_ALMOST_DONE"=FALSE, "OUT_AUXILIARY"=FALSE, "OUT_SERIAL_DATA"=FALSE, "IN_TRIGGER_ENABLE"=TRUE, "IN_DIGITAL_TRIGGER"=TRUE, "IN_GATE"=FALSE, "IN_CAPTURE_ON_DEMAND"=FALSE, "IN_RESET_TIMESTAMP"=FALSE, "IN_SLOW_EXTERNAL_CLOCK"=FALSE, "INPUT_AUXILIARY"=FALSE, "INPUT_SERIAL_DATA"=FALSE}, "ChannelsPerBoard"=2}}, {"Name"="ATS9325", "Specifications"={"ClckSource"={"Internal"=TRUE, "External"=TRUE, "Medium Ext."=FALSE, "Slow Ext."=TRUE, "Ext. AC"=FALSE, "Ext. DC"=FALSE, "Ext. (PLL)"=TRUE}, "ClckRate"={"1 kS/s"=TRUE, "2 kS/s"=TRUE, "5 kS/s"=TRUE, "10 kS/s"=TRUE, "20 kS/s"=TRUE, "50 kS/s"=TRUE, "100 kS/s"=TRUE, "200 kS/s"=TRUE, "500 kS/s"=TRUE, "1 MS/s"=TRUE, "2 MS/s"=TRUE, "5 MS/s"=TRUE, "10 MS/s"=TRUE, "20 MS/s"=TRUE, "25 MS/s"=FALSE, "50 MS/s"=TRUE, "100 MS/s"=TRUE, "125 MS/s"=FALSE, "160 MS/s"=FALSE, "180 MS/s"=FALSE, "200 MS/s"=FALSE, "250 MS/s"=TRUE, "500 MS/s"=FALSE, "1 GS/s"=FALSE}, "ClckEdge"={"Rising"=TRUE, "Falling"=TRUE}, "InputCoupling"={"AC"=TRUE, "DC"=TRUE}, "InputRange"={"20mV"=FALSE, "40mV"=TRUE, "50mV"=FALSE, "80mV"=FALSE, "100mV"=TRUE, "200mV"=TRUE, "400mV"=TRUE, "500mV"=FALSE, "800mV"=FALSE, "1 V"=TRUE, "2 V"=TRUE, "4 V"=TRUE, "5 V"=FALSE, "8 V"=FALSE, "10 V"=FALSE, "16 V"=FALSE, "20 V"=FALSE, "40 V"=FALSE, "HiFi"=FALSE, "1.25 V"=FALSE}, "Impedance"={"1M ohms"=FALSE, "50 ohms"=TRUE, "300 ohms"=FALSE}, "Bandwidth"={"Full"=TRUE, "Reduce"=FALSE}, "RangeLim(50)"="4 V", "AsyncDMA"={"OnBoard"=TRUE, "FPGA"=FALSE}, "Memory"={"VerifMem"=FALSE, "HighMem"=TRUE, "Combine"=FALSE, "HighRecord"=TRUE}, "ExtTrigCoupling"={"AC"=TRUE, "DC"=TRUE}, "ExtTrigRange"={"1 V"=TRUE, "5 V"=TRUE, "\nTTL"=FALSE}, "AUX_IO_Trig"={"Trig_Out"=TRUE, "Trig_In"=TRUE}, "AUX_IO_Slope"={"Rising"=TRUE, "Falling"=TRUE}, "MaxPretrig"={"MEM"=0, "FIFO"=0}, "AUX_I/O_Trig"={"OUT_Trigger"=TRUE, "OUT_PACER"=FALSE, "OUT_BUSY"=FALSE, "OUT_CLOCK"=FALSE, "OUT_RESERVED"=FALSE, "OUT_CAPTURE_ALMOST_DONE"=FALSE, "OUT_AUXILIARY"=FALSE, "OUT_SERIAL_DATA"=FALSE, "IN_TRIGGER_ENABLE"=TRUE, "IN_DIGITAL_TRIGGER"=TRUE, "IN_GATE"=FALSE, "IN_CAPTURE_ON_DEMAND"=FALSE, "IN_RESET_TIMESTAMP"=FALSE, "IN_SLOW_EXTERNAL_CLOCK"=FALSE, "INPUT_AUXILIARY"=FALSE, "INPUT_SERIAL_DATA"=FALSE}, "ChannelsPerBoard"=2}}, {"Name"="ATS9440", "Specifications"={"ClckSource"={"Internal"=TRUE, "External"=TRUE, "Medium Ext."=TRUE, "Slow Ext."=TRUE, "Ext. AC"=FALSE, "Ext. DC"=FALSE, "Ext. (PLL)"=TRUE}, "ClckRate"={"1 kS/s"=FALSE, "2 kS/s"=FALSE, "5 kS/s"=FALSE, "10 kS/s"=TRUE, "20 kS/s"=TRUE, "50 kS/s"=TRUE, "100 kS/s"=TRUE, "200 kS/s"=TRUE, "500 kS/s"=TRUE, "1 MS/s"=TRUE, "2 MS/s"=TRUE, "5 MS/s"=TRUE, "10 MS/s"=TRUE, "20 MS/s"=TRUE, "25 MS/s"=FALSE, "50 MS/s"=TRUE, "100 MS/s"=TRUE, "125 MS/s"=TRUE, "160 MS/s"=FALSE, "180 MS/s"=FALSE, "200 MS/s"=FALSE, "250 MS/s"=FALSE, "500 MS/s"=FALSE, "1 GS/s"=FALSE}, "ClckEdge"={"Rising"=TRUE, "Falling"=TRUE}, "InputCoupling"={"AC"=FALSE, "DC"=TRUE}, "InputRange"={"20mV"=FALSE, "40mV"=FALSE, "50mV"=FALSE, "80mV"=FALSE, "100mV"=TRUE, "200mV"=TRUE, "400mV"=TRUE, "500mV"=FALSE, "800mV"=FALSE, "1 V"=TRUE, "2 V"=TRUE, "4 V"=TRUE, "5 V"=FALSE, "8 V"=FALSE, "10 V"=FALSE, "16 V"=FALSE, "20 V"=FALSE, "40 V"=FALSE, "HiFi"=FALSE, "1.25 V"=FALSE}, "Impedance"={"1M ohms"=FALSE, "50 ohms"=TRUE, "300 ohms"=FALSE}, "Bandwidth"={"Full"=TRUE, "Reduce"=FALSE}, "RangeLim(50)"="4 V", "AsyncDMA"={"OnBoard"=TRUE, "FPGA"=TRUE}, "Memory"={"VerifMem"=FALSE, "HighMem"=TRUE, "Combine"=FALSE, "HighRecord"=TRUE}, "ExtTrigCoupling"={"AC"=TRUE, "DC"=TRUE}, "ExtTrigRange"={"1 V"=FALSE, "5 V"=TRUE, "\nTTL"=FALSE}, "AUX_IO_Trig"={"Trig_Out"=TRUE, "Trig_In"=TRUE}, "AUX_IO_Slope"={"Rising"=TRUE, "Falling"=TRUE}, "MaxPretrig"={"MEM"=0, "FIFO"=0}, "AUX_I/O_Trig"={"OUT_Trigger"=TRUE, "OUT_PACER"=FALSE, "OUT_BUSY"=FALSE, "OUT_CLOCK"=FALSE, "OUT_RESERVED"=FALSE, "OUT_CAPTURE_ALMOST_DONE"=FALSE, "OUT_AUXILIARY"=FALSE, "OUT_SERIAL_DATA"=FALSE, "IN_TRIGGER_ENABLE"=TRUE, "IN_DIGITAL_TRIGGER"=TRUE, "IN_GATE"=FALSE, "IN_CAPTURE_ON_DEMAND"=FALSE, "IN_RESET_TIMESTAMP"=FALSE, "IN_SLOW_EXTERNAL_CLOCK"=FALSE, "INPUT_AUXILIARY"=FALSE, "INPUT_SERIAL_DATA"=FALSE}, "ChannelsPerBoard"=4}}, {"Name"="ATS9410\nATS9410", "Specifications"={"ClckSource"={"Internal"=TRUE, "External"=TRUE, "Medium Ext."=TRUE, "Slow Ext."=TRUE, "Ext. AC"=FALSE, "Ext. DC"=FALSE, "Ext. (PLL)"=TRUE}, "ClckRate"={"1 kS/s"=FALSE, "2 kS/s"=FALSE, "5 kS/s"=FALSE, "10 kS/s"=TRUE, "20 kS/s"=TRUE, "50 kS/s"=TRUE, "100 kS/s"=TRUE, "200 kS/s"=TRUE, "500 kS/s"=TRUE, "1 MS/s"=TRUE, "2 MS/s"=TRUE, "5 MS/s"=TRUE, "10 MS/s"=TRUE, "20 MS/s"=TRUE, "25 MS/s"=FALSE, "50 MS/s"=TRUE, "100 MS/s"=TRUE, "125 MS/s"=TRUE, "160 MS/s"=FALSE, "180 MS/s"=FALSE, "200 MS/s"=FALSE, "250 MS/s"=FALSE, "500 MS/s"=FALSE, "1 GS/s"=FALSE}, "ClckEdge"={"Rising"=TRUE, "Falling"=TRUE}, "InputCoupling"={"AC"=FALSE, "DC"=TRUE}, "InputRange"={"20mV"=FALSE, "40mV"=FALSE, "50mV"=FALSE, "80mV"=FALSE, "100mV"=TRUE, "200mV"=TRUE, "400mV"=TRUE, "500mV"=FALSE, "800mV"=FALSE, "1 V"=TRUE, "2 V"=TRUE, "4 V"=TRUE, "5 V"=FALSE, "8 V"=FALSE, "10 V"=FALSE, "16 V"=FALSE, "20 V"=FALSE, "40 V"=FALSE, "HiFi"=FALSE, "1.25 V"=FALSE}, "Impedance"={"1M ohms"=FALSE, "50 ohms"=TRUE, "300 ohms"=FALSE}, "Bandwidth"={"Full"=TRUE, "Reduce"=FALSE}, "RangeLim(50)"="4 V", "AsyncDMA"={"OnBoard"=TRUE, "FPGA"=TRUE}, "Memory"={"VerifMem"=FALSE, "HighMem"=TRUE, "Combine"=FALSE, "HighRecord"=TRUE}, "ExtTrigCoupling"={"AC"=TRUE, "DC"=TRUE}, "ExtTrigRange"={"1 V"=FALSE, "5 V"=TRUE, "\nTTL"=FALSE}, "AUX_IO_Trig"={"Trig_Out"=TRUE, "Trig_In"=TRUE}, "AUX_IO_Slope"={"Rising"=TRUE, "Falling"=TRUE}, "MaxPretrig"={"MEM"=0, "FIFO"=0}, "AUX_I/O_Trig"={"OUT_Trigger"=TRUE, "OUT_PACER"=FALSE, "OUT_BUSY"=FALSE, "OUT_CLOCK"=FALSE, "OUT_RESERVED"=FALSE, "OUT_CAPTURE_ALMOST_DONE"=FALSE, "OUT_AUXILIARY"=FALSE, "OUT_SERIAL_DATA"=FALSE, "IN_TRIGGER_ENABLE"=TRUE, "IN_DIGITAL_TRIGGER"=TRUE, "IN_GATE"=FALSE, "IN_CAPTURE_ON_DEMAND"=FALSE, "IN_RESET_TIMESTAMP"=FALSE, "IN_SLOW_EXTERNAL_CLOCK"=FALSE, "INPUT_AUXILIARY"=FALSE, "INPUT_SERIAL_DATA"=FALSE}, "ChannelsPerBoard"=2}}, {"Name"="ATS9351", "Specifications"={"ClckSource"={"Internal"=TRUE, "External"=TRUE, "Medium Ext."=FALSE, "Slow Ext."=TRUE, "Ext. AC"=FALSE, "Ext. DC"=FALSE, "Ext. (PLL)"=TRUE}, "ClckRate"={"1 kS/s"=TRUE, "2 kS/s"=TRUE, "5 kS/s"=TRUE, "10 kS/s"=TRUE, "20 kS/s"=TRUE, "50 kS/s"=TRUE, "100 kS/s"=TRUE, "200 kS/s"=TRUE, "500 kS/s"=TRUE, "1 MS/s"=TRUE, "2 MS/s"=TRUE, "5 MS/s"=TRUE, "10 MS/s"=TRUE, "20 MS/s"=TRUE, "25 MS/s"=FALSE, "50 MS/s"=TRUE, "100 MS/s"=TRUE, "125 MS/s"=FALSE, "160 MS/s"=FALSE, "180 MS/s"=FALSE, "200 MS/s"=FALSE, "250 MS/s"=TRUE, "500 MS/s"=TRUE, "1 GS/s"=FALSE}, "ClckEdge"={"Rising"=TRUE, "Falling"=TRUE}, "InputCoupling"={"AC"=TRUE, "DC"=TRUE}, "InputRange"={"20mV"=FALSE, "40mV"=FALSE, "50mV"=FALSE, "80mV"=FALSE, "100mV"=FALSE, "200mV"=FALSE, "400mV"=TRUE, "500mV"=FALSE, "800mV"=FALSE, "1 V"=FALSE, "2 V"=FALSE, "4 V"=FALSE, "5 V"=FALSE, "8 V"=FALSE, "10 V"=FALSE, "16 V"=FALSE, "20 V"=FALSE, "40 V"=FALSE, "HiFi"=FALSE, "1.25 V"=FALSE}, "Impedance"={"1M ohms"=FALSE, "50 ohms"=TRUE, "300 ohms"=FALSE}, "Bandwidth"={"Full"=TRUE, "Reduce"=FALSE}, "RangeLim(50)"="4 V", "AsyncDMA"={"OnBoard"=TRUE, "FPGA"=FALSE}, "Memory"={"VerifMem"=FALSE, "HighMem"=TRUE, "Combine"=FALSE, "HighRecord"=TRUE}, "ExtTrigCoupling"={"AC"=TRUE, "DC"=TRUE}, "ExtTrigRange"={"1 V"=FALSE, "5 V"=TRUE, "\nTTL"=FALSE}, "AUX_IO_Trig"={"Trig_Out"=TRUE, "Trig_In"=TRUE}, "AUX_IO_Slope"={"Rising"=TRUE, "Falling"=TRUE}, "MaxPretrig"={"MEM"=0, "FIFO"=0}, "AUX_I/O_Trig"={"OUT_Trigger"=TRUE, "OUT_PACER"=FALSE, "OUT_BUSY"=FALSE, "OUT_CLOCK"=FALSE, "OUT_RESERVED"=FALSE, "OUT_CAPTURE_ALMOST_DONE"=FALSE, "OUT_AUXILIARY"=FALSE, "OUT_SERIAL_DATA"=FALSE, "IN_TRIGGER_ENABLE"=TRUE, "IN_DIGITAL_TRIGGER"=TRUE, "IN_GATE"=FALSE, "IN_CAPTURE_ON_DEMAND"=FALSE, "IN_RESET_TIMESTAMP"=FALSE, "IN_SLOW_EXTERNAL_CLOCK"=FALSE, "INPUT_AUXILIARY"=FALSE, "INPUT_SERIAL_DATA"=FALSE}, "ChannelsPerBoard"=2}}, {"Name"="ATS9310", "Specifications"={"ClckSource"={"Internal"=TRUE, "External"=TRUE, "Medium Ext."=FALSE, "Slow Ext."=FALSE, "Ext. AC"=FALSE, "Ext. DC"=FALSE, "Ext. (PLL)"=TRUE}, "ClckRate"={"1 kS/s"=TRUE, "2 kS/s"=TRUE, "5 kS/s"=TRUE, "10 kS/s"=TRUE, "20 kS/s"=TRUE, "50 kS/s"=TRUE, "100 kS/s"=TRUE, "200 kS/s"=TRUE, "500 kS/s"=TRUE, "1 MS/s"=TRUE, "2 MS/s"=TRUE, "5 MS/s"=TRUE, "10 MS/s"=TRUE, "20 MS/s"=TRUE, "25 MS/s"=FALSE, "50 MS/s"=TRUE, "100 MS/s"=TRUE, "125 MS/s"=FALSE, "160 MS/s"=FALSE, "180 MS/s"=FALSE, "200 MS/s"=FALSE, "250 MS/s"=FALSE, "500 MS/s"=FALSE, "1 GS/s"=FALSE}, "ClckEdge"={"Rising"=TRUE, "Falling"=TRUE}, "InputCoupling"={"AC"=TRUE, "DC"=TRUE}, "InputRange"={"20mV"=FALSE, "40mV"=TRUE, "50mV"=FALSE, "80mV"=FALSE, "100mV"=TRUE, "200mV"=TRUE, "400mV"=TRUE, "500mV"=FALSE, "800mV"=FALSE, "1 V"=TRUE, "2 V"=TRUE, "4 V"=TRUE, "5 V"=FALSE, "8 V"=FALSE, "10 V"=FALSE, "16 V"=FALSE, "20 V"=FALSE, "40 V"=FALSE, "HiFi"=FALSE, "1.25 V"=FALSE}, "Impedance"={"1M ohms"=FALSE, "50 ohms"=TRUE, "300 ohms"=FALSE}, "Bandwidth"={"Full"=TRUE, "Reduce"=FALSE}, "RangeLim(50)"="4 V", "AsyncDMA"={"OnBoard"=TRUE, "FPGA"=FALSE}, "Memory"={"VerifMem"=FALSE, "HighMem"=TRUE, "Combine"=FALSE, "HighRecord"=TRUE}, "ExtTrigCoupling"={"AC"=TRUE, "DC"=TRUE}, "ExtTrigRange"={"1 V"=FALSE, "5 V"=TRUE, "\nTTL"=FALSE}, "AUX_IO_Trig"={"Trig_Out"=TRUE, "Trig_In"=TRUE}, "AUX_IO_Slope"={"Rising"=TRUE, "Falling"=TRUE}, "MaxPretrig"={"MEM"=0, "FIFO"=0}, "AUX_I/O_Trig"={"OUT_Trigger"=TRUE, "OUT_PACER"=FALSE, "OUT_BUSY"=FALSE, "OUT_CLOCK"=FALSE, "OUT_RESERVED"=FALSE, "OUT_CAPTURE_ALMOST_DONE"=FALSE, "OUT_AUXILIARY"=FALSE, "OUT_SERIAL_DATA"=FALSE, "IN_TRIGGER_ENABLE"=TRUE, "IN_DIGITAL_TRIGGER"=TRUE, "IN_GATE"=FALSE, "IN_CAPTURE_ON_DEMAND"=FALSE, "IN_RESET_TIMESTAMP"=FALSE, "IN_SLOW_EXTERNAL_CLOCK"=FALSE, "INPUT_AUXILIARY"=FALSE, "INPUT_SERIAL_DATA"=FALSE}, "ChannelsPerBoard"=2}}, {"Name"="ATS9461", "Specifications"={"ClckSource"={"Internal"=TRUE, "External"=TRUE, "Medium Ext."=FALSE, "Slow Ext."=TRUE, "Ext. AC"=FALSE, "Ext. DC"=TRUE, "Ext. (PLL)"=TRUE}, "ClckRate"={"1 kS/s"=TRUE, "2 kS/s"=TRUE, "5 kS/s"=TRUE, "10 kS/s"=TRUE, "20 kS/s"=TRUE, "50 kS/s"=TRUE, "100 kS/s"=TRUE, "200 kS/s"=TRUE, "500 kS/s"=TRUE, "1 MS/s"=TRUE, "2 MS/s"=TRUE, "5 MS/s"=TRUE, "10 MS/s"=TRUE, "20 MS/s"=TRUE, "25 MS/s"=FALSE, "50 MS/s"=TRUE, "100 MS/s"=TRUE, "125 MS/s"=TRUE, "160 MS/s"=TRUE, "180 MS/s"=TRUE, "200 MS/s"=FALSE, "250 MS/s"=FALSE, "500 MS/s"=FALSE, "1 GS/s"=FALSE}, "ClckEdge"={"Rising"=TRUE, "Falling"=TRUE}, "InputCoupling"={"AC"=TRUE, "DC"=TRUE}, "InputRange"={"20mV"=FALSE, "40mV"=FALSE, "50mV"=FALSE, "80mV"=FALSE, "100mV"=FALSE, "200mV"=TRUE, "400mV"=TRUE, "500mV"=FALSE, "800mV"=TRUE, "1 V"=FALSE, "2 V"=TRUE, "4 V"=TRUE, "5 V"=FALSE, "8 V"=TRUE, "10 V"=FALSE, "16 V"=TRUE, "20 V"=FALSE, "40 V"=FALSE, "HiFi"=FALSE, "1.25 V"=FALSE}, "Impedance"={"1M ohms"=TRUE, "50 ohms"=TRUE, "300 ohms"=FALSE}, "Bandwidth"={"Full"=TRUE, "Reduce"=TRUE}, "RangeLim(50)"="4 V", "AsyncDMA"={"OnBoard"=TRUE, "FPGA"=TRUE}, "Memory"={"VerifMem"=FALSE, "HighMem"=TRUE, "Combine"=FALSE, "HighRecord"=TRUE}, "ExtTrigCoupling"={"AC"=TRUE, "DC"=TRUE}, "ExtTrigRange"={"1 V"=TRUE, "5 V"=TRUE, "\nTTL"=FALSE}, "AUX_IO_Trig"={"Trig_Out"=TRUE, "Trig_In"=TRUE}, "AUX_IO_Slope"={"Rising"=TRUE, "Falling"=TRUE}, "MaxPretrig"={"MEM"=0, "FIFO"=0}, "AUX_I/O_Trig"={"OUT_Trigger"=TRUE, "OUT_PACER"=FALSE, "OUT_BUSY"=FALSE, "OUT_CLOCK"=FALSE, "OUT_RESERVED"=FALSE, "OUT_CAPTURE_ALMOST_DONE"=FALSE, "OUT_AUXILIARY"=FALSE, "OUT_SERIAL_DATA"=FALSE, "IN_TRIGGER_ENABLE"=TRUE, "IN_DIGITAL_TRIGGER"=TRUE, "IN_GATE"=FALSE, "IN_CAPTURE_ON_DEMAND"=FALSE, "IN_RESET_TIMESTAMP"=FALSE, "IN_SLOW_EXTERNAL_CLOCK"=FALSE, "INPUT_AUXILIARY"=FALSE, "INPUT_SERIAL_DATA"=FALSE}, "ChannelsPerBoard"=2}}, {"Name"="ATS9850", "Specifications"={"ClckSource"={"Internal"=TRUE, "External"=FALSE, "Medium Ext."=FALSE, "Slow Ext."=FALSE, "Ext. AC"=TRUE, "Ext. DC"=TRUE, "Ext. (PLL)"=TRUE}, "ClckRate"={"1 kS/s"=TRUE, "2 kS/s"=TRUE, "5 kS/s"=TRUE, "10 kS/s"=TRUE, "20 kS/s"=TRUE, "50 kS/s"=TRUE, "100 kS/s"=TRUE, "200 kS/s"=TRUE, "500 kS/s"=TRUE, "1 MS/s"=TRUE, "2 MS/s"=TRUE, "5 MS/s"=TRUE, "10 MS/s"=TRUE, "20 MS/s"=TRUE, "25 MS/s"=FALSE, "50 MS/s"=TRUE, "100 MS/s"=TRUE, "125 MS/s"=FALSE, "160 MS/s"=FALSE, "180 MS/s"=FALSE, "200 MS/s"=FALSE, "250 MS/s"=TRUE, "500 MS/s"=TRUE, "1 GS/s"=FALSE}, "ClckEdge"={"Rising"=TRUE, "Falling"=TRUE}, "InputCoupling"={"AC"=TRUE, "DC"=TRUE}, "InputRange"={"20mV"=FALSE, "40mV"=FALSE, "50mV"=FALSE, "80mV"=FALSE, "100mV"=FALSE, "200mV"=TRUE, "400mV"=TRUE, "500mV"=FALSE, "800mV"=FALSE, "1 V"=TRUE, "2 V"=TRUE, "4 V"=TRUE, "5 V"=FALSE, "8 V"=FALSE, "10 V"=FALSE, "16 V"=FALSE, "20 V"=FALSE, "40 V"=FALSE, "HiFi"=FALSE, "1.25 V"=FALSE}, "Impedance"={"1M ohms"=FALSE, "50 ohms"=TRUE, "300 ohms"=FALSE}, "Bandwidth"={"Full"=TRUE, "Reduce"=FALSE}, "RangeLim(50)"="4 V", "AsyncDMA"={"OnBoard"=TRUE, "FPGA"=TRUE}, "Memory"={"VerifMem"=FALSE, "HighMem"=TRUE, "Combine"=FALSE, "HighRecord"=TRUE}, "ExtTrigCoupling"={"AC"=TRUE, "DC"=TRUE}, "ExtTrigRange"={"1 V"=FALSE, "5 V"=TRUE, "\nTTL"=FALSE}, "AUX_IO_Trig"={"Trig_Out"=TRUE, "Trig_In"=TRUE}, "AUX_IO_Slope"={"Rising"=TRUE, "Falling"=TRUE}, "MaxPretrig"={"MEM"=268433408, "FIFO"=0}, "AUX_I/O_Trig"={"OUT_Trigger"=TRUE, "OUT_PACER"=FALSE, "OUT_BUSY"=FALSE, "OUT_CLOCK"=FALSE, "OUT_RESERVED"=FALSE, "OUT_CAPTURE_ALMOST_DONE"=FALSE, "OUT_AUXILIARY"=FALSE, "OUT_SERIAL_DATA"=FALSE, "IN_TRIGGER_ENABLE"=TRUE, "IN_DIGITAL_TRIGGER"=TRUE, "IN_GATE"=FALSE, "IN_CAPTURE_ON_DEMAND"=FALSE, "IN_RESET_TIMESTAMP"=FALSE, "IN_SLOW_EXTERNAL_CLOCK"=FALSE, "INPUT_AUXILIARY"=FALSE, "INPUT_SERIAL_DATA"=FALSE}, "ChannelsPerBoard"=2}}, {"Name"="ATS9625", "Specifications"={"ClckSource"={"Internal"=TRUE, "External"=FALSE, "Medium Ext."=FALSE, "Slow Ext."=TRUE, "Ext. AC"=TRUE, "Ext. DC"=FALSE, "Ext. (PLL)"=TRUE}, "ClckRate"={"1 kS/s"=TRUE, "2 kS/s"=TRUE, "5 kS/s"=TRUE, "10 kS/s"=TRUE, "20 kS/s"=TRUE, "50 kS/s"=TRUE, "100 kS/s"=TRUE, "200 kS/s"=TRUE, "500 kS/s"=TRUE, "1 MS/s"=TRUE, "2 MS/s"=TRUE, "5 MS/s"=TRUE, "10 MS/s"=TRUE, "20 MS/s"=TRUE, "25 MS/s"=FALSE, "50 MS/s"=TRUE, "100 MS/s"=TRUE, "125 MS/s"=TRUE, "160 MS/s"=FALSE, "180 MS/s"=FALSE, "200 MS/s"=TRUE, "250 MS/s"=TRUE, "500 MS/s"=FALSE, "1 GS/s"=FALSE}, "ClckEdge"={"Rising"=TRUE, "Falling"=TRUE}, "InputCoupling"={"AC"=TRUE, "DC"=FALSE}, "InputRange"={"20mV"=FALSE, "40mV"=FALSE, "50mV"=FALSE, "80mV"=FALSE, "100mV"=FALSE, "200mV"=FALSE, "400mV"=FALSE, "500mV"=FALSE, "800mV"=FALSE, "1 V"=FALSE, "2 V"=FALSE, "4 V"=FALSE, "5 V"=FALSE, "8 V"=FALSE, "10 V"=FALSE, "16 V"=FALSE, "20 V"=FALSE, "40 V"=FALSE, "HiFi"=FALSE, "1.25 V"=TRUE}, "Impedance"={"1M ohms"=FALSE, "50 ohms"=TRUE, "300 ohms"=FALSE}, "Bandwidth"={"Full"=TRUE, "Reduce"=FALSE}, "RangeLim(50)"="1.25", "AsyncDMA"={"OnBoard"=TRUE, "FPGA"=FALSE}, "Memory"={"VerifMem"=FALSE, "HighMem"=TRUE, "Combine"=FALSE, "HighRecord"=TRUE}, "ExtTrigCoupling"={"AC"=TRUE, "DC"=TRUE}, "ExtTrigRange"={"1 V"=FALSE, "5 V"=TRUE, "\nTTL"=TRUE}, "AUX_IO_Trig"={"Trig_Out"=TRUE, "Trig_In"=TRUE}, "AUX_IO_Slope"={"Rising"=TRUE, "Falling"=TRUE}, "MaxPretrig"={"MEM"=2147481600, "FIFO"=0}, "AUX_I/O_Trig"={"OUT_Trigger"=TRUE, "OUT_PACER"=FALSE, "OUT_BUSY"=FALSE, "OUT_CLOCK"=FALSE, "OUT_RESERVED"=FALSE, "OUT_CAPTURE_ALMOST_DONE"=FALSE, "OUT_AUXILIARY"=FALSE, "OUT_SERIAL_DATA"=FALSE, "IN_TRIGGER_ENABLE"=TRUE, "IN_DIGITAL_TRIGGER"=TRUE, "IN_GATE"=FALSE, "IN_CAPTURE_ON_DEMAND"=FALSE, "IN_RESET_TIMESTAMP"=FALSE, "IN_SLOW_EXTERNAL_CLOCK"=FALSE, "INPUT_AUXILIARY"=FALSE, "INPUT_SERIAL_DATA"=FALSE}, "ChannelsPerBoard"=2}}, {"Name"="ATG6500", "Specifications"={"ClckSource"={"Internal"=FALSE, "External"=FALSE, "Medium Ext."=FALSE, "Slow Ext."=FALSE, "Ext. AC"=FALSE, "Ext. DC"=FALSE, "Ext. (PLL)"=FALSE}, "ClckRate"={"1 kS/s"=FALSE, "2 kS/s"=FALSE, "5 kS/s"=FALSE, "10 kS/s"=FALSE, "20 kS/s"=FALSE, "50 kS/s"=FALSE, "100 kS/s"=FALSE, "200 kS/s"=FALSE, "500 kS/s"=FALSE, "1 MS/s"=FALSE, "2 MS/s"=FALSE, "5 MS/s"=FALSE, "10 MS/s"=FALSE, "20 MS/s"=FALSE, "25 MS/s"=FALSE, "50 MS/s"=FALSE, "100 MS/s"=FALSE, "125 MS/s"=FALSE, "160 MS/s"=FALSE, "180 MS/s"=FALSE, "200 MS/s"=FALSE, "250 MS/s"=FALSE, "500 MS/s"=FALSE, "1 GS/s"=FALSE}, "ClckEdge"={"Rising"=FALSE, "Falling"=FALSE}, "InputCoupling"={"AC"=FALSE, "DC"=TRUE}, "InputRange"={"20mV"=FALSE, "40mV"=FALSE, "50mV"=FALSE, "80mV"=FALSE, "100mV"=FALSE, "200mV"=FALSE, "400mV"=FALSE, "500mV"=FALSE, "800mV"=FALSE, "1 V"=FALSE, "2 V"=FALSE, "4 V"=FALSE, "5 V"=FALSE, "8 V"=FALSE, "10 V"=FALSE, "16 V"=FALSE, "20 V"=FALSE, "40 V"=FALSE, "HiFi"=FALSE, "1.25 V"=FALSE}, "Impedance"={"1M ohms"=FALSE, "50 ohms"=FALSE, "300 ohms"=FALSE}, "Bandwidth"={"Full"=FALSE, "Reduce"=FALSE}, "RangeLim(50)"="4", "AsyncDMA"={"OnBoard"=FALSE, "FPGA"=FALSE}, "Memory"={"VerifMem"=FALSE, "HighMem"=FALSE, "Combine"=FALSE, "HighRecord"=FALSE}, "ExtTrigCoupling"={"AC"=FALSE, "DC"=TRUE}, "ExtTrigRange"={"1 V"=FALSE, "5 V"=FALSE, "\nTTL"=TRUE}, "AUX_IO_Trig"={"Trig_Out"=FALSE, "Trig_In"=FALSE}, "AUX_IO_Slope"={"Rising"=FALSE, "Falling"=FALSE}, "MaxPretrig"={"MEM"=0, "FIFO"=0}, "AUX_I/O_Trig"={"OUT_Trigger"=FALSE, "OUT_PACER"=FALSE, "OUT_BUSY"=FALSE, "OUT_CLOCK"=FALSE, "OUT_RESERVED"=FALSE, "OUT_CAPTURE_ALMOST_DONE"=FALSE, "OUT_AUXILIARY"=FALSE, "OUT_SERIAL_DATA"=FALSE, "IN_TRIGGER_ENABLE"=FALSE, "IN_DIGITAL_TRIGGER"=FALSE, "IN_GATE"=FALSE, "IN_CAPTURE_ON_DEMAND"=FALSE, "IN_RESET_TIMESTAMP"=FALSE, "IN_SLOW_EXTERNAL_CLOCK"=FALSE, "INPUT_AUXILIARY"=FALSE, "INPUT_SERIAL_DATA"=FALSE}, "ChannelsPerBoard"=2}}, {"Name"="ATS9626", "Specifications"={"ClckSource"={"Internal"=TRUE, "External"=FALSE, "Medium Ext."=FALSE, "Slow Ext."=TRUE, "Ext. AC"=TRUE, "Ext. DC"=FALSE, "Ext. (PLL)"=TRUE}, "ClckRate"={"1 kS/s"=TRUE, "2 kS/s"=TRUE, "5 kS/s"=TRUE, "10 kS/s"=TRUE, "20 kS/s"=TRUE, "50 kS/s"=TRUE, "100 kS/s"=TRUE, "200 kS/s"=TRUE, "500 kS/s"=TRUE, "1 MS/s"=TRUE, "2 MS/s"=TRUE, "5 MS/s"=TRUE, "10 MS/s"=TRUE, "20 MS/s"=TRUE, "25 MS/s"=FALSE, "50 MS/s"=TRUE, "100 MS/s"=TRUE, "125 MS/s"=TRUE, "160 MS/s"=FALSE, "180 MS/s"=FALSE, "200 MS/s"=FALSE, "250 MS/s"=TRUE, "500 MS/s"=FALSE, "1 GS/s"=FALSE}, "ClckEdge"={"Rising"=TRUE, "Falling"=TRUE}, "InputCoupling"={"AC"=FALSE, "DC"=TRUE}, "InputRange"={"20mV"=FALSE, "40mV"=FALSE, "50mV"=FALSE, "80mV"=FALSE, "100mV"=FALSE, "200mV"=FALSE, "400mV"=FALSE, "500mV"=FALSE, "800mV"=FALSE, "1 V"=FALSE, "2 V"=FALSE, "4 V"=FALSE, "5 V"=FALSE, "8 V"=FALSE, "10 V"=FALSE, "16 V"=FALSE, "20 V"=FALSE, "40 V"=FALSE, "HiFi"=FALSE, "1.25 V"=TRUE}, "Impedance"={"1M ohms"=FALSE, "50 ohms"=TRUE, "300 ohms"=FALSE}, "Bandwidth"={"Full"=TRUE, "Reduce"=FALSE}, "RangeLim(50)"="1.25", "AsyncDMA"={"OnBoard"=TRUE, "FPGA"=FALSE}, "Memory"={"VerifMem"=FALSE, "HighMem"=TRUE, "Combine"=FALSE, "HighRecord"=TRUE}, "ExtTrigCoupling"={"AC"=TRUE, "DC"=TRUE}, "ExtTrigRange"={"1 V"=FALSE, "5 V"=TRUE, "\nTTL"=TRUE}, "AUX_IO_Trig"={"Trig_Out"=TRUE, "Trig_In"=TRUE}, "AUX_IO_Slope"={"Rising"=FALSE, "Falling"=FALSE}, "MaxPretrig"={"MEM"=134215680, "FIFO"=0}, "AUX_I/O_Trig"={"OUT_Trigger"=TRUE, "OUT_PACER"=FALSE, "OUT_BUSY"=FALSE, "OUT_CLOCK"=FALSE, "OUT_RESERVED"=FALSE, "OUT_CAPTURE_ALMOST_DONE"=FALSE, "OUT_AUXILIARY"=FALSE, "OUT_SERIAL_DATA"=FALSE, "IN_TRIGGER_ENABLE"=TRUE, "IN_DIGITAL_TRIGGER"=TRUE, "IN_GATE"=FALSE, "IN_CAPTURE_ON_DEMAND"=FALSE, "IN_RESET_TIMESTAMP"=FALSE, "IN_SLOW_EXTERNAL_CLOCK"=FALSE, "INPUT_AUXILIARY"=FALSE, "INPUT_SERIAL_DATA"=FALSE}, "ChannelsPerBoard"=2}}]
  in  "Cards_Pre-Set":T2[](array[typedef])=[{"Record"={"Count"=1, "Presize"=512, "Length"=4096}, "Clock"={"ClckSource"=enum."Internal", "ClckRate"=14, "ClckEdge"=0, "Decimation"=0}, "Inputs"=[{"Coupling"=enum."DC", "Range"=9, "Impedance"=enum."1M ohms", "Bandwidth"=enum."Full Bandwidth"}, {"Coupling"=enum."DC", "Range"=9, "Impedance"=enum."1M ohms", "Bandwidth"=enum."Full Bandwidth"}], "Trigger"={"TrigOperation"=enum."Only X", "Timeout (s)"=1.0, "Trig. Delay"=0, "Engine X"={"Source"=enum."Chan_A", "Slope"=enum."Positive", "Level"=128}, "Engine Y"={"Source"=enum."Disable", "Slope"=enum."Positive", "Level"=128}, "ExtTrigControl"={"Coupling"=enum."AC", "Range"=enum."1 V"}}}, {"Record"={"Count"=1, "Presize"=512, "Length"=4096}, "Clock"={"ClckSource"=enum."Internal", "ClckRate"=14, "ClckEdge"=0, "Decimation"=0}, "Inputs"=[{"Coupling"=enum."DC", "Range"=9, "Impedance"=enum."1M ohms", "Bandwidth"=enum."Full Bandwidth"}, {"Coupling"=enum."DC", "Range"=9, "Impedance"=enum."1M ohms", "Bandwidth"=enum."Full Bandwidth"}], "Trigger"={"TrigOperation"=enum."Only X", "Timeout (s)"=1.0, "Trig. Delay"=0, "Engine X"={"Source"=enum."Chan_A", "Slope"=enum."Positive", "Level"=128}, "Engine Y"={"Source"=enum."Disable", "Slope"=enum."Positive", "Level"=128}, "ExtTrigControl"={"Coupling"=enum."AC", "Range"=enum."1 V"}}}, {"Record"={"Count"=1, "Presize"=512, "Length"=4096}, "Clock"={"ClckSource"=enum."Internal", "ClckRate"=13, "ClckEdge"=0, "Decimation"=0}, "Inputs"=[{"Coupling"=enum."DC", "Range"=8, "Impedance"=enum."1M ohms", "Bandwidth"=enum."Full Bandwidth"}, {"Coupling"=enum."DC", "Range"=8, "Impedance"=enum."1M ohms", "Bandwidth"=enum."Full Bandwidth"}], "Trigger"={"TrigOperation"=enum."Only X", "Timeout (s)"=1.0, "Trig. Delay"=0, "Engine X"={"Source"=enum."Chan_A", "Slope"=enum."Positive", "Level"=128}, "Engine Y"={"Source"=enum."Disable", "Slope"=enum."Positive", "Level"=128}, "ExtTrigControl"={"Coupling"=enum."AC", "Range"=enum."1 V"}}}, {"Record"={"Count"=1, "Presize"=512, "Length"=4096}, "Clock"={"ClckSource"=enum."Internal", "ClckRate"=14, "ClckEdge"=0, "Decimation"=0}, "Inputs"=[{"Coupling"=enum."DC", "Range"=8, "Impedance"=enum."1M ohms", "Bandwidth"=enum."Full Bandwidth"}, {"Coupling"=enum."DC", "Range"=8, "Impedance"=enum."1M ohms", "Bandwidth"=enum."Full Bandwidth"}], "Trigger"={"TrigOperation"=enum."Only X", "Timeout (s)"=1.0, "Trig. Delay"=0, "Engine X"={"Source"=enum."Chan_A", "Slope"=enum."Positive", "Level"=128}, "Engine Y"={"Source"=enum."Disable", "Slope"=enum."Positive", "Level"=128}, "ExtTrigControl"={"Coupling"=enum."AC", "Range"=enum."1 V"}}}, {"Record"={"Count"=0, "Presize"=0, "Length"=0}, "Clock"={"ClckSource"=enum."Internal", "ClckRate"=13, "ClckEdge"=0, "Decimation"=0}, "Inputs"=[{"Coupling"=enum."AC", "Range"=9, "Impedance"=enum."1M ohms", "Bandwidth"=enum."Full Bandwidth"}, {"Coupling"=enum."AC", "Range"=9, "Impedance"=enum."1M ohms", "Bandwidth"=enum."Full Bandwidth"}], "Trigger"={"TrigOperation"=enum."Only X", "Timeout (s)"=1.0, "Trig. Delay"=0, "Engine X"={"Source"=enum."Chan_A", "Slope"=enum."Positive", "Level"=128}, "Engine Y"={"Source"=enum."Disable", "Slope"=enum."Positive", "Level"=128}, "ExtTrigControl"={"Coupling"=enum."AC", "Range"=enum."1 V"}}}, {"Record"={"Count"=0, "Presize"=0, "Length"=0}, "Clock"={"ClckSource"=enum."Internal", "ClckRate"=13, "ClckEdge"=0, "Decimation"=0}, "Inputs"=[{"Coupling"=enum."AC", "Range"=9, "Impedance"=enum."1M ohms", "Bandwidth"=enum."Full Bandwidth"}, {"Coupling"=enum."AC", "Range"=9, "Impedance"=enum."1M ohms", "Bandwidth"=enum."Full Bandwidth"}], "Trigger"={"TrigOperation"=enum."Only X", "Timeout (s)"=1.0, "Trig. Delay"=0, "Engine X"={"Source"=enum."Chan_A", "Slope"=enum."Positive", "Level"=128}, "Engine Y"={"Source"=enum."Disable", "Slope"=enum."Positive", "Level"=128}, "ExtTrigControl"={"Coupling"=enum."AC", "Range"=enum."1 V"}}}, {"Record"={"Count"=1, "Presize"=512, "Length"=4096}, "Clock"={"ClckSource"=enum."Internal", "ClckRate"=13, "ClckEdge"=0, "Decimation"=0}, "Inputs"=[{"Coupling"=enum."DC", "Range"=9, "Impedance"=enum."1M ohms", "Bandwidth"=enum."Full Bandwidth"}, {"Coupling"=enum."DC", "Range"=9, "Impedance"=enum."1M ohms", "Bandwidth"=enum."Full Bandwidth"}], "Trigger"={"TrigOperation"=enum."Only X", "Timeout (s)"=1.0, "Trig. Delay"=0, "Engine X"={"Source"=enum."Chan_A", "Slope"=enum."Positive", "Level"=128}, "Engine Y"={"Source"=enum."Disable", "Slope"=enum."Positive", "Level"=128}, "ExtTrigControl"={"Coupling"=enum."AC", "Range"=enum."1 V"}}}, {"Record"={"Count"=1, "Presize"=512, "Length"=4096}, "Clock"={"ClckSource"=enum."Internal", "ClckRate"=16, "ClckEdge"=0, "Decimation"=0}, "Inputs"=[{"Coupling"=enum."DC", "Range"=2, "Impedance"=enum."1M ohms", "Bandwidth"=enum."Full Bandwidth"}, {"Coupling"=enum."DC", "Range"=2, "Impedance"=enum."1M ohms", "Bandwidth"=enum."Full Bandwidth"}], "Trigger"={"TrigOperation"=enum."Only X", "Timeout (s)"=1.0, "Trig. Delay"=0, "Engine X"={"Source"=enum."Chan_A", "Slope"=enum."Positive", "Level"=128}, "Engine Y"={"Source"=enum."Disable", "Slope"=enum."Positive", "Level"=128}, "ExtTrigControl"={"Coupling"=enum."AC", "Range"=enum."1 V"}}}, {"Record"={"Count"=1, "Presize"=512, "Length"=4096}, "Clock"={"ClckSource"=enum."Internal", "ClckRate"=16, "ClckEdge"=0, "Decimation"=0}, "Inputs"=[{"Coupling"=enum."DC", "Range"=8, "Impedance"=enum."1M ohms", "Bandwidth"=enum."Full Bandwidth"}, {"Coupling"=enum."DC", "Range"=8, "Impedance"=enum."1M ohms", "Bandwidth"=enum."Full Bandwidth"}], "Trigger"={"TrigOperation"=enum."Only X", "Timeout (s)"=1.0, "Trig. Delay"=0, "Engine X"={"Source"=enum."Chan_A", "Slope"=enum."Positive", "Level"=128}, "Engine Y"={"Source"=enum."Disable", "Slope"=enum."Positive", "Level"=128}, "ExtTrigControl"={"Coupling"=enum."AC", "Range"=enum."1 V"}}}, {"Record"={"Count"=1, "Presize"=512, "Length"=4096}, "Clock"={"ClckSource"=enum."Internal", "ClckRate"=16, "ClckEdge"=0, "Decimation"=0}, "Inputs"=[{"Coupling"=enum."DC", "Range"=2, "Impedance"=enum."1M ohms", "Bandwidth"=enum."Full Bandwidth"}, {"Coupling"=enum."DC", "Range"=2, "Impedance"=enum."1M ohms", "Bandwidth"=enum."Full Bandwidth"}], "Trigger"={"TrigOperation"=enum."Only X", "Timeout (s)"=1.0, "Trig. Delay"=0, "Engine X"={"Source"=enum."Chan_A", "Slope"=enum."Positive", "Level"=128}, "Engine Y"={"Source"=enum."Disable", "Slope"=enum."Positive", "Level"=128}, "ExtTrigControl"={"Coupling"=enum."AC", "Range"=enum."1 V"}}}, {"Record"={"Count"=1, "Presize"=512, "Length"=4096}, "Clock"={"ClckSource"=enum."Internal", "ClckRate"=16, "ClckEdge"=0, "Decimation"=0}, "Inputs"=[{"Coupling"=enum."DC", "Range"=2, "Impedance"=enum."1M ohms", "Bandwidth"=enum."Full Bandwidth"}, {"Coupling"=enum."DC", "Range"=2, "Impedance"=enum."1M ohms", "Bandwidth"=enum."Full Bandwidth"}], "Trigger"={"TrigOperation"=enum."Only X", "Timeout (s)"=1.0, "Trig. Delay"=0, "Engine X"={"Source"=enum."Chan_A", "Slope"=enum."Positive", "Level"=128}, "Engine Y"={"Source"=enum."Disable", "Slope"=enum."Positive", "Level"=128}, "ExtTrigControl"={"Coupling"=enum."AC", "Range"=enum."1 V"}}}, {"Record"={"Count"=1, "Presize"=0, "Length"=4096}, "Clock"={"ClckSource"=enum."Internal", "ClckRate"=18, "ClckEdge"=0, "Decimation"=0}, "Inputs"=[{"Coupling"=enum."DC", "Range"=2, "Impedance"=enum."1M ohms", "Bandwidth"=enum."Full Bandwidth"}, {"Coupling"=enum."DC", "Range"=2, "Impedance"=enum."1M ohms", "Bandwidth"=enum."Full Bandwidth"}], "Trigger"={"TrigOperation"=enum."Only X", "Timeout (s)"=1.0, "Trig. Delay"=0, "Engine X"={"Source"=enum."Chan_A", "Slope"=enum."Positive", "Level"=128}, "Engine Y"={"Source"=enum."Disable", "Slope"=enum."Positive", "Level"=128}, "ExtTrigControl"={"Coupling"=enum."AC", "Range"=enum."1 V"}}}, {"Record"={"Count"=1, "Presize"=512, "Length"=4096}, "Clock"={"ClckSource"=enum."Internal", "ClckRate"=16, "ClckEdge"=0, "Decimation"=0}, "Inputs"=[{"Coupling"=enum."DC", "Range"=2, "Impedance"=enum."1M ohms", "Bandwidth"=enum."Full Bandwidth"}, {"Coupling"=enum."DC", "Range"=2, "Impedance"=enum."1M ohms", "Bandwidth"=enum."Full Bandwidth"}], "Trigger"={"TrigOperation"=enum."Only X", "Timeout (s)"=1.0, "Trig. Delay"=0, "Engine X"={"Source"=enum."Chan_A", "Slope"=enum."Positive", "Level"=128}, "Engine Y"={"Source"=enum."Disable", "Slope"=enum."Positive", "Level"=128}, "ExtTrigControl"={"Coupling"=enum."AC", "Range"=enum."1 V"}}}, {"Record"={"Count"=1, "Presize"=512, "Length"=4096}, "Clock"={"ClckSource"=enum."Internal", "ClckRate"=18, "ClckEdge"=0, "Decimation"=0}, "Inputs"=[{"Coupling"=enum."DC", "Range"=2, "Impedance"=enum."50 ohms", "Bandwidth"=enum."Full Bandwidth"}, {"Coupling"=enum."DC", "Range"=2, "Impedance"=enum."50 ohms", "Bandwidth"=enum."Full Bandwidth"}], "Trigger"={"TrigOperation"=enum."Only X", "Timeout (s)"=1.0, "Trig. Delay"=0, "Engine X"={"Source"=enum."Chan_A", "Slope"=enum."Positive", "Level"=128}, "Engine Y"={"Source"=enum."Disable", "Slope"=enum."Positive", "Level"=128}, "ExtTrigControl"={"Coupling"=enum."AC", "Range"=enum."1 V"}}}, {"Record"={"Count"=1, "Presize"=512, "Length"=4096}, "Clock"={"ClckSource"=enum."Internal", "ClckRate"=19, "ClckEdge"=0, "Decimation"=0}, "Inputs"=[{"Coupling"=enum."DC", "Range"=4, "Impedance"=enum."50 ohms", "Bandwidth"=enum."Full Bandwidth"}, {"Coupling"=enum."DC", "Range"=4, "Impedance"=enum."50 ohms", "Bandwidth"=enum."Full Bandwidth"}], "Trigger"={"TrigOperation"=enum."Only X", "Timeout (s)"=1.0, "Trig. Delay"=0, "Engine X"={"Source"=enum."Chan_A", "Slope"=enum."Positive", "Level"=128}, "Engine Y"={"Source"=enum."Disable", "Slope"=enum."Positive", "Level"=128}, "ExtTrigControl"={"Coupling"=enum."DC", "Range"=enum."5 V"}}}, {"Record"={"Count"=1, "Presize"=512, "Length"=4096}, "Clock"={"ClckSource"=enum."Internal", "ClckRate"=16, "ClckEdge"=0, "Decimation"=0}, "Inputs"=[{"Coupling"=enum."DC", "Range"=4, "Impedance"=enum."50 ohms", "Bandwidth"=enum."Full Bandwidth"}, {"Coupling"=enum."DC", "Range"=4, "Impedance"=enum."50 ohms", "Bandwidth"=enum."Full Bandwidth"}], "Trigger"={"TrigOperation"=enum."Only X", "Timeout (s)"=1.0, "Trig. Delay"=0, "Engine X"={"Source"=enum."Chan_A", "Slope"=enum."Positive", "Level"=128}, "Engine Y"={"Source"=enum."Disable", "Slope"=enum."Positive", "Level"=128}, "ExtTrigControl"={"Coupling"=enum."DC", "Range"=enum."5 V"}}}, {"Record"={"Count"=1, "Presize"=512, "Length"=4096}, "Clock"={"ClckSource"=enum."Internal", "ClckRate"=13, "ClckEdge"=0, "Decimation"=0}, "Inputs"=[{"Coupling"=enum."DC", "Range"=3, "Impedance"=enum."50 ohms", "Bandwidth"=enum."Full Bandwidth"}, {"Coupling"=enum."DC", "Range"=3, "Impedance"=enum."50 ohms", "Bandwidth"=enum."Full Bandwidth"}, {"Coupling"=enum."DC", "Range"=3, "Impedance"=enum."50 ohms", "Bandwidth"=enum."Full Bandwidth"}, {"Coupling"=enum."DC", "Range"=3, "Impedance"=enum."50 ohms", "Bandwidth"=enum."Full Bandwidth"}], "Trigger"={"TrigOperation"=enum."Only X", "Timeout (s)"=1.0, "Trig. Delay"=0, "Engine X"={"Source"=enum."Chan_A", "Slope"=enum."Positive", "Level"=128}, "Engine Y"={"Source"=enum."Disable", "Slope"=enum."Positive", "Level"=128}, "ExtTrigControl"={"Coupling"=enum."AC", "Range"=enum."5 V"}}}, {"Record"={"Count"=1, "Presize"=512, "Length"=4096}, "Clock"={"ClckSource"=enum."Internal", "ClckRate"=16, "ClckEdge"=0, "Decimation"=0}, "Inputs"=[{"Coupling"=enum."DC", "Range"=9, "Impedance"=enum."1M ohms", "Bandwidth"=enum."Full Bandwidth"}, {"Coupling"=enum."DC", "Range"=9, "Impedance"=enum."1M ohms", "Bandwidth"=enum."Full Bandwidth"}], "Trigger"={"TrigOperation"=enum."Only X", "Timeout (s)"=1.0, "Trig. Delay"=0, "Engine X"={"Source"=enum."Chan_A", "Slope"=enum."Positive", "Level"=128}, "Engine Y"={"Source"=enum."Disable", "Slope"=enum."Positive", "Level"=128}, "ExtTrigControl"={"Coupling"=enum."AC", "Range"=enum."5 V"}}}, {"Record"={"Count"=1, "Presize"=512, "Length"=4096}, "Clock"={"ClckSource"=enum."Internal", "ClckRate"=16, "ClckEdge"=0, "Decimation"=0}, "Inputs"=[{"Coupling"=enum."DC", "Range"=9, "Impedance"=enum."1M ohms", "Bandwidth"=enum."Full Bandwidth"}, {"Coupling"=enum."DC", "Range"=9, "Impedance"=enum."1M ohms", "Bandwidth"=enum."Full Bandwidth"}], "Trigger"={"TrigOperation"=enum."Only X", "Timeout (s)"=1.0, "Trig. Delay"=0, "Engine X"={"Source"=enum."Chan_A", "Slope"=enum."Positive", "Level"=128}, "Engine Y"={"Source"=enum."Disable", "Slope"=enum."Positive", "Level"=128}, "ExtTrigControl"={"Coupling"=enum."DC", "Range"=enum."5 V"}}}, {"Record"={"Count"=1, "Presize"=512, "Length"=4096}, "Clock"={"ClckSource"=enum."Internal", "ClckRate"=16, "ClckEdge"=0, "Decimation"=0}, "Inputs"=[{"Coupling"=enum."DC", "Range"=9, "Impedance"=enum."1M ohms", "Bandwidth"=enum."Full Bandwidth"}, {"Coupling"=enum."DC", "Range"=9, "Impedance"=enum."1M ohms", "Bandwidth"=enum."Full Bandwidth"}], "Trigger"={"TrigOperation"=enum."Only X", "Timeout (s)"=1.0, "Trig. Delay"=0, "Engine X"={"Source"=enum."Chan_A", "Slope"=enum."Positive", "Level"=128}, "Engine Y"={"Source"=enum."Disable", "Slope"=enum."Positive", "Level"=128}, "ExtTrigControl"={"Coupling"=enum."AC", "Range"=enum."5 V"}}}, {"Record"={"Count"=1, "Presize"=512, "Length"=4096}, "Clock"={"ClckSource"=enum."Internal", "ClckRate"=16, "ClckEdge"=0, "Decimation"=0}, "Inputs"=[{"Coupling"=enum."DC", "Range"=9, "Impedance"=enum."1M ohms", "Bandwidth"=enum."Full Bandwidth"}, {"Coupling"=enum."DC", "Range"=9, "Impedance"=enum."1M ohms", "Bandwidth"=enum."Full Bandwidth"}], "Trigger"={"TrigOperation"=enum."Only X", "Timeout (s)"=1.0, "Trig. Delay"=0, "Engine X"={"Source"=enum."Chan_A", "Slope"=enum."Positive", "Level"=128}, "Engine Y"={"Source"=enum."Disable", "Slope"=enum."Positive", "Level"=128}, "ExtTrigControl"={"Coupling"=enum."AC", "Range"=enum."5 V"}}}, {"Record"={"Count"=1, "Presize"=512, "Length"=4096}, "Clock"={"ClckSource"=enum."Internal", "ClckRate"=13, "ClckEdge"=0, "Decimation"=0}, "Inputs"=[{"Coupling"=enum."DC", "Range"=9, "Impedance"=enum."50 ohms", "Bandwidth"=enum."Full Bandwidth"}, {"Coupling"=enum."DC", "Range"=9, "Impedance"=enum."50 ohms", "Bandwidth"=enum."Full Bandwidth"}], "Trigger"={"TrigOperation"=enum."Only X", "Timeout (s)"=1.0, "Trig. Delay"=0, "Engine X"={"Source"=enum."Chan_A", "Slope"=enum."Positive", "Level"=128}, "Engine Y"={"Source"=enum."Disable", "Slope"=enum."Positive", "Level"=128}, "ExtTrigControl"={"Coupling"=enum."DC", "Range"=enum."5 V"}}}, {"Record"={"Count"=1, "Presize"=512, "Length"=4096}, "Clock"={"ClckSource"=enum."Internal", "ClckRate"=19, "ClckEdge"=0, "Decimation"=0}, "Inputs"=[{"Coupling"=enum."AC", "Range"=10, "Impedance"=enum."50 ohms", "Bandwidth"=enum."Full Bandwidth"}, {"Coupling"=enum."AC", "Range"=10, "Impedance"=enum."50 ohms", "Bandwidth"=enum."Full Bandwidth"}], "Trigger"={"TrigOperation"=enum."Only X", "Timeout (s)"=1.0, "Trig. Delay"=0, "Engine X"={"Source"=enum."External", "Slope"=enum."Positive", "Level"=140}, "Engine Y"={"Source"=enum."Disable", "Slope"=enum."Positive", "Level"=128}, "ExtTrigControl"={"Coupling"=enum."DC", "Range"=enum."5 V"}}}, {"Record"={"Count"=1, "Presize"=512, "Length"=4096}, "Clock"={"ClckSource"=enum."Internal", "ClckRate"=19, "ClckEdge"=0, "Decimation"=0}, "Inputs"=[{"Coupling"=enum."DC", "Range"=9, "Impedance"=enum."1M ohms", "Bandwidth"=enum."Full Bandwidth"}, {"Coupling"=enum."DC", "Range"=9, "Impedance"=enum."1M ohms", "Bandwidth"=enum."Full Bandwidth"}], "Trigger"={"TrigOperation"=enum."Only X", "Timeout (s)"=1.0, "Trig. Delay"=0, "Engine X"={"Source"=enum."Chan_A", "Slope"=enum."Positive", "Level"=128}, "Engine Y"={"Source"=enum."Disable", "Slope"=enum."Positive", "Level"=128}, "ExtTrigControl"={"Coupling"=enum."AC", "Range"=enum."5 V"}}}, {"Record"={"Count"=1, "Presize"=512, "Length"=4096}, "Clock"={"ClckSource"=enum."Internal", "ClckRate"=19, "ClckEdge"=0, "Decimation"=0}, "Inputs"=[{"Coupling"=enum."DC", "Range"=10, "Impedance"=enum."50 ohms", "Bandwidth"=enum."Full Bandwidth"}, {"Coupling"=enum."DC", "Range"=10, "Impedance"=enum."50 ohms", "Bandwidth"=enum."Full Bandwidth"}], "Trigger"={"TrigOperation"=enum."Only X", "Timeout (s)"=1.0, "Trig. Delay"=0, "Engine X"={"Source"=enum."External", "Slope"=enum."Positive", "Level"=140}, "Engine Y"={"Source"=enum."Disable", "Slope"=enum."Positive", "Level"=128}, "ExtTrigControl"={"Coupling"=enum."AC", "Range"=enum."5 V"}}}] {"Inputs"."Range" items=["20mV", "40mV", "50mV", "80mV", "100mV", "200mV", "400mV", "500mV", "800mV", "1 V", "1.25 V", "2 V", "4 V", "5 V", "8 V", "10 V", "16 V", "20 V", "40 V", "HiFi"]; "Clock"."ClckEdge" items=["Rising", "Falling"]; "Clock"."ClckRate" items=["1 kS/s", "2 kS/s", "5 kS/s", "10 kS/s", "20 kS/s", "50 kS/s", "100 kS/s", "200 kS/s", "500 kS/s", "1 MS/s", "2 MS/s", "5 MS/s", "10 MS/s", "20 MS/s", "25 MS/s", "50 MS/s", "100 MS/s", "125 MS/s", "200 MS/s", "250 MS/s", "500 MS/s", "1 GS/s"]; "Trigger"."Timeout (s)" format="%.2f"}
  in  "Cards_Specs":T20[](array[typedef])=[{"Name"="Unknown", "Rate"=["1 kS/s", "2 kS/s", "5 kS/s", "10 kS/s", "20 kS/s", "50 kS/s", "100 kS/s", "200 kS/s", "500 kS/s", "1 MS/s", "2 MS/s", "5 MS/s", "10 MS/s", "20 MS/s", "25 MS/s", "50 MS/s", "100 MS/s", "200 MS/s", "500 MS/s", "1 GS/s"], "Range"=["20mv", "40mV", "50mV", "80mV", "100mV", "200mV", "400mV", "500mV", "800mV", "1 V", "2 V", "4 V", "5 V", "8 V", "10 V", "20 V"], "RangeLim(50)"=15, "Bandwidth"=FALSE}, {"Name"="ATS850", "Rate"=["1 kS/s", "2 kS/s", "5 kS/s", "10 kS/s", "20 kS/s", "50 kS/s", "100 kS/s", "200 kS/s", "500 kS/s", "1 MS/s", "2 MS/s", "5 MS/s", "10 MS/s", "25 MS/s", "50 MS/s"], "Range"=["20mv", "40mV", "50mV", "80mV", "100mV", "200mV", "400mV", "500mV", "800mV", "1 V", "2 V", "4 V", "5 V", "8 V", "10 V", "20 V"], "RangeLim(50)"=15, "Bandwidth"=FALSE}, {"Name"="ATS310", "Rate"=["1 kS/s", "2 kS/s", "5 kS/s", "10 kS/s", "20 kS/s", "50 kS/s", "100 kS/s", "200 kS/s", "500 kS/s", "1 MS/s", "2 MS/s", "5 MS/s", "10 MS/s", "20 MS/s"], "Range"=["40mV", "50mV", "80mV", "100mV", "200mV", "400mV", "500mV", "800mV", "1 V", "2 V", "4 V", "5 V", "8 V", "10 V", "20 V"], "RangeLim(50)"=10, "Bandwidth"=FALSE}, {"Name"="ATS330", "Rate"=["1 kS/s", "2 kS/s", "5 kS/s", "10 kS/s", "20 kS/s", "50 kS/s", "100 kS/s", "200 kS/s", "500 kS/s", "1 MS/s", "2 MS/s", "5 MS/s", "10 MS/s", "25 MS/s", "50 MS/s"], "Range"=["40mV", "50mV", "80mV", "100mV", "200mV", "400mV", "500mV", "800mV", "1 V", "2 V", "4 V", "5 V", "8 V", "10 V", "20 V"], "RangeLim(50)"=10, "Bandwidth"=FALSE}, {"Name"="ATSxx4", "Rate"=["1 kS/s", "2 kS/s", "5 kS/s", "10 kS/s", "20 kS/s", "50 kS/s", "100 kS/s", "200 kS/s", "500 kS/s", "1 MS/s", "2 MS/s", "5 MS/s", "10 MS/s", "20 MS/s", "25 MS/s", "50 MS/s", "100 MS/s", "200 MS/s", "500 MS/s", "1 GS/s"], "Range"=["20mv", "40mV", "50mV", "80mV", "100mV", "200mV", "400mV", "500mV", "800mV", "1 V", "2 V", "4 V", "5 V", "8 V", "10 V", "20 V"], "RangeLim(50)"=15, "Bandwidth"=FALSE}, {"Name"="ATSxx5", "Rate"=["1 kS/s", "2 kS/s", "5 kS/s", "10 kS/s", "20 kS/s", "50 kS/s", "100 kS/s", "200 kS/s", "500 kS/s", "1 MS/s", "2 MS/s", "5 MS/s", "10 MS/s", "20 MS/s", "25 MS/s", "50 MS/s", "100 MS/s", "200 MS/s", "500 MS/s", "1 GS/s"], "Range"=["20mv", "40mV", "50mV", "80mV", "100mV", "200mV", "400mV", "500mV", "800mV", "1 V", "2 V", "4 V", "5 V", "8 V", "10 V", "20 V"], "RangeLim(50)"=15, "Bandwidth"=FALSE}, {"Name"="ATS460", "Rate"=["10 kS/s", "20 kS/s", "50 kS/s", "100 kS/s", "200 kS/s", "500 kS/s", "1 MS/s", "2 MS/s", "5 MS/s", "10 MS/s", "20 MS/s", "50 MS/s", "100 MS/s", "125 MS/s"], "Range"=["20mV", "40mV", "50mV", "80mV", "100mV", "200mV", "400mV", "500mV", "800mV", "1 V", "2 V", "4 V", "5 V", "8 V", "10 V", "HiFi"], "RangeLim(50)"=11, "Bandwidth"=TRUE}, {"Name"="ATS660", "Rate"=["1 kS/s", "2 kS/s", "5 kS/s", "10 kS/s", "20 kS/s", "50 kS/s", "100 kS/s", "200 kS/s", "500 kS/s", "1 MS/s", "2 MS/s", "5 MS/s", "10 MS/s", "20 MS/s", "50 MS/s", "100 MS/s", "125 MS/s"], "Range"=["200mV", "400mV", "800mV", "2 V", "4 V", "8 V", "16 V"], "RangeLim(50)"=4, "Bandwidth"=TRUE}, {"Name"="ATS860", "Rate"=["1 kS/s", "2 kS/s", "5 kS/s", "10 kS/s", "20 kS/s", "50 kS/s", "100 kS/s", "200 kS/s", "500 kS/s", "1 MS/s", "2 MS/s", "5 MS/s", "10 MS/s", "25 MS/s", "50 MS/s", "125 MS/s", "250 MS/s"], "Range"=["20mV", "50mV", "80mV", "100mV", "200mV", "400mV", "500mV", "800mV", "1 V", "2 V", "4 V", "5 V", "8 V", "10 V"], "RangeLim(50)"=10, "Bandwidth"=TRUE}, {"Name"="UNKNOWN", "Rate"=["1 kS/s", "2 kS/s", "5 kS/s", "10 kS/s", "20 kS/s", "50 kS/s", "100 kS/s", "200 kS/s", "500 kS/s", "1 MS/s", "2 MS/s", "5 MS/s", "10 MS/s", "20 MS/s", "50 MS/s", "100 MS/s", "125 MS/s"], "Range"=["200mV", "400mV", "800mV", "2 V", "4 V", "8 V", "16 V"], "RangeLim(50)"=4, "Bandwidth"=TRUE}, {"Name"="UNKNOWN", "Rate"=["1 kS/s", "2 kS/s", "5 kS/s", "10 kS/s", "20 kS/s", "50 kS/s", "100 kS/s", "200 kS/s", "500 kS/s", "1 MS/s", "2 MS/s", "5 MS/s", "10 MS/s", "20 MS/s", "50 MS/s", "100 MS/s", "125 MS/s"], "Range"=["200mV", "400mV", "800mV", "2 V", "4 V", "8 V", "16 V"], "RangeLim(50)"=4, "Bandwidth"=TRUE}, {"Name"="ATS9462", "Rate"=["1 kS/s", "2 kS/s", "5 kS/s", "10 kS/s", "20 kS/s", "50 kS/s", "100 kS/s", "200 kS/s", "500 kS/s", "1 MS/s", "2 MS/s", "5 MS/s", "10 MS/s", "20 MS/s", "50 MS/s", "100 MS/s", "125 MS/s", "160 MS/s", "180 MS/s"], "Range"=["200mV", "400mV", "800mV", "2 V", "4 V", "8 V", "16 V"], "RangeLim(50)"=4, "Bandwidth"=TRUE}]
  # "IMPORTANT:  In the \"Cards_Pre-Set\" array the \"name\" in the ring selectors is not important,  only the value in the Digital display\nis use to select the value (rate or range) from the corresponding array in the \"Cards_Specs\""
  # "<==To keep for compatibility"
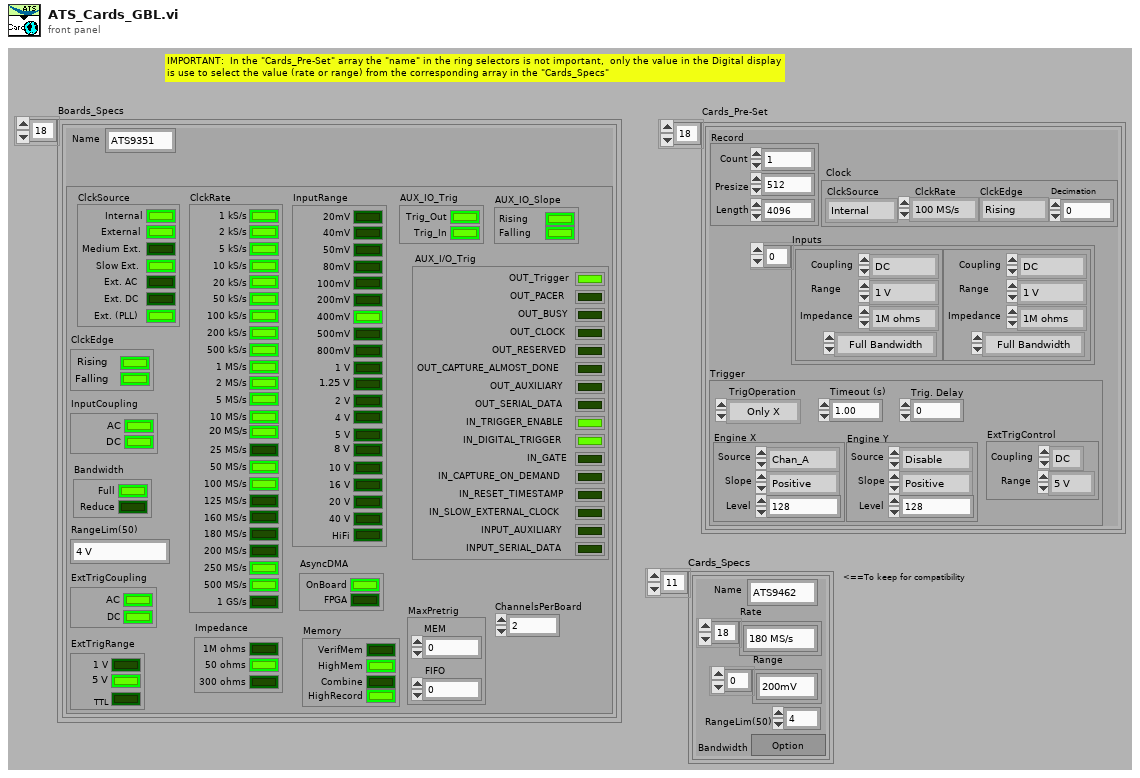
[diagram p1: front panel]
types:
  T1 = typedef "ATS_Global_Specs_Ctrl.ctl" = cluster{"ClckSource":cluster{"Internal":bool, "External":bool, "Medium Ext.":bool, "Slow Ext.":bool, "Ext. AC":bool, "Ext. DC":bool, "Ext. (PLL)":bool}, "ClckRate":cluster{"1 kS/s":bool, "2 kS/s":bool, "5 kS/s":bool, "10 kS/s":bool, "20 kS/s":bool, "50 kS/s":bool, "100 kS/s":bool, "200 kS/s":bool, "500 kS/s":bool, "1 MS/s":bool, "2 MS/s":bool, "5 MS/s":bool, "10 MS/s":bool, "20 MS/s":bool, "25 MS/s":bool, "50 MS/s":bool, "100 MS/s":bool, "125 MS/s":bool, "160 MS/s":bool, "180 MS/s":bool, "200 MS/s":bool, "250 MS/s":bool, "500 MS/s":bool, "1 GS/s":bool}, "ClckEdge":cluster{"Rising":bool, "Falling":bool}, "InputCoupling":cluster{"AC":bool, "DC":bool}, "InputRange":cluster{"20mV":bool, "40mV":bool, "50mV":bool, "80mV":bool, "100mV":bool, "200mV":bool, "400mV":bool, "500mV":bool, "800mV":bool, "1 V":bool, "2 V":bool, "4 V":bool, "5 V":bool, "8 V":bool, "10 V":bool, "16 V":bool, "20 V":bool, "40 V":bool, "HiFi":bool, "1.25 V":bool}, "Impedance":cluster{"1M ohms":bool, "50 ohms":bool, "300 ohms":bool}, "Bandwidth":cluster{"Full":bool, "Reduce":bool}, "RangeLim(50)":string, "AsyncDMA":cluster{"OnBoard":bool, "FPGA":bool}, "Memory":cluster{"VerifMem":bool, "HighMem":bool, "Combine":bool, "HighRecord":bool}, "ExtTrigCoupling":cluster{"AC":bool, "DC":bool}, "ExtTrigRange":cluster{"1 V":bool, "5 V":bool, "\nTTL":bool}, "AUX_IO_Trig":cluster{"Trig_Out":bool, "Trig_In":bool}, "AUX_IO_Slope":cluster{"Rising":bool, "Falling":bool}, "MaxPretrig":cluster{"MEM":u32, "FIFO":u32}, "AUX_I/O_Trig":cluster{"OUT_Trigger":bool, "OUT_PACER":bool, "OUT_BUSY":bool, "OUT_CLOCK":bool, "OUT_RESERVED":bool, "OUT_CAPTURE_ALMOST_DONE":bool, "OUT_AUXILIARY":bool, "OUT_SERIAL_DATA":bool, "IN_TRIGGER_ENABLE":bool, "IN_DIGITAL_TRIGGER":bool, "IN_GATE":bool, "IN_CAPTURE_ON_DEMAND":bool, "IN_RESET_TIMESTAMP":bool, "IN_SLOW_EXTERNAL_CLOCK":bool, "INPUT_AUXILIARY":bool, "INPUT_SERIAL_DATA":bool}, "ChannelsPerBoard":u8}
  T2 = typedef "ATS_Global_4Ch.ctl" = cluster{"Record":T3, "Clock":T4, "Inputs":T8, "Trigger":T14}
  T3 = typedef "Record.ctl" = cluster{"Count":u32, "Presize":u32, "Length":u32}
  T4 = typedef "Clock.ctl" = cluster{"ClckSource":T5, "ClckRate":T6, "ClckEdge":T7, "Decimation":u32}
  T5 = typedef "ClockSource.ctl" = enum16{"Internal", "External", "Medium Ext.", "Slow Ext.", "Ext. AC", "Ext. DC", "Ext. (PLL)"}
  T6 = typedef "ClockRate.ctl" = u32
  T7 = typedef "ClockEdge.ctl" = u16
  T8 = typedef "ATS_InputArray.ctl" = T9[]
  T9 = typedef "InputCtrl.ctl" = cluster{"Coupling":T10, "Range":T11, "Impedance":T12, "Bandwidth":T13}
  T10 = typedef "Coupling.ctl" = enum16{"AC", "DC"}
  T11 = typedef "Range.ctl" = u32
  T12 = typedef "Impedance.ctl" = enum16{"1M ohms", "50 ohms"}
  T13 = typedef "Bandwidth.ctl" = enum16{"Full Bandwidth", "Reduce Bandwidth"}
  T14 = typedef "ATS_Trigger_4Ch.ctl" = cluster{"TrigOperation":T15, "Timeout (s)":dbl, "Trig. Delay":u32, "Engine X":T16, "Engine Y":T16, "ExtTrigControl":T18}
  T15 = typedef "TriggerOperation.ctl" = enum16{"Only X", "Only Y", "X or Y", "X and Y", "X xor Y", "X and not Y", "not X and Y"}
  T16 = typedef "ATS_TriggerEngine_4Ch.ctl" = cluster{"Source":T17, "Slope":enum32{"Positive", "Negative"}, "Level":u32}
  T17 = typedef "ATS_TriggerSource_4Ch.ctl" = enum32{"Chan_A", "Chan_B", "External", "Disable", "Chan_C", "Chan_D"}
  T18 = typedef "ExtTrigger.ctl" = cluster{"Coupling":T10, "Range":T19}
  T19 = typedef "ExtTrigRange.ctl" = enum16{"1 V", "5 V", "TTL"}
  T20 = typedef "ATS_Card_Spec.ctl" = cluster{"Name":string, "Rate":string[], "Range":string[], "RangeLim(50)":u32, "Bandwidth":bool}
diagram:
